vi "FFT Analysis (V1.24) 1.vi"() -> ()   [LabVIEW 2020]
uses:
  API/Generic Utilities_class/Generic Utilities.lvclass
  gSPWB.lvclass
  <vilib>/addons/_AddQ/G#Object/G#Object.lvclass
  API/GSwFormDSP_class/GSwFormDSP.lvclass
  API/GSwFormDSP_class/functions/Spectrum Display Options.ctl
  API/GSwFormDSP_class/functions/Attribute List.ctl
  C:/Program Files/National Instruments/LabVIEW 2020/vi.lib/addons/_AddQ/G#Object/G#Object.lvclass
  C:/Program Files/National Instruments/LabVIEW 2020/vi.lib/addons/_AddQ/IG#/IG#.lvclass
  C:/Users/fcharett/docsWork/coding/20openSourceSPWB/API/Generic Utilities_class/Generic Utilities.lvclass
  C:/Users/fcharett/docsWork/coding/20openSourceSPWB/API/GSwFormDSP_class/GSwFormDSP.lvclass
  SPWB.lvclass
  C:/Users/fcharett/docsWork/coding/20openSourceSPWB/SPWB_class/SPWB.lvclass
  API/GSwFormDSP_class/functions/Spectral Function Type.ctl
  <vilib>/Analysis/4window.llb/windowTd.ctl
  <vilib>/Analysis/NI_AALPro.lvlib
  API/GSwFormDSP_class/functions/Acoustic Weighting.ctl
panel:
  out "Version":string
  in  "Plot Names":string[](array[string])
  in  "Help":bool
  in  "wForms":waveform(dbl)[](array[waveform])
  in  "Exit":bool
  in  "reference in":refnum<class "SPWB.lvclass">
  out "PSD":waveform(dbl)[](array[waveform])
  in  "Signals selector":bool[](array[boolean])
  in  "DSP Functions":T1(tab)=enum."Spectral Analysis"
  in  "Load FROM File:":T2(ring)
  in  "Acoustic Weighting":T3
  in  "Spectrum Display Options":T4
  in  "Spectral Function Type":T5
  in  "Spectral Function Parameters - User":T7={"Frequency resolution (Hz)"=enum."1.0 Hz", "Overlap in %"=enum."0", "Window"=0} {"Window" items=["Rectangle"=0, "Hanning"=1, "Hamming"=2, "Blackman-Harris"=3, "Exact Blackman"=4, "Blackman"=5, "Flat Top"=6, "4 Term B-Harris "=7, "7 Term B-Harris"=8, "Low Sidelobe"=9, "Blackman Nuttall"=11, "Triangle"=30, "Bartlett-Hanning"=31, "Bohman"=32, "Parzen"=33, "Welch"=34, "Kaiser"=60, "Dolph-Chebyshev"=61, "Gaussian"=62]}
  in  "Average":enum16{"Select Here ...", "Energetic Average"}(ring)
  in  "Integrate":bool
  in  "Differentiate":bool
  in  "End Frequency (Hz)":dbl
  out "EB Result Table":string[][](table)
  in  "Start Frequency (Hz)":dbl
  in  "Export table to clipboard":bool
  in  "Import Signals":u16(ring) items=["Import Signals from another figure ..."]
  in  "Delete signals":bool
  in  "Graph":waveform(dbl)[](graph) caption="Waveform Graph"
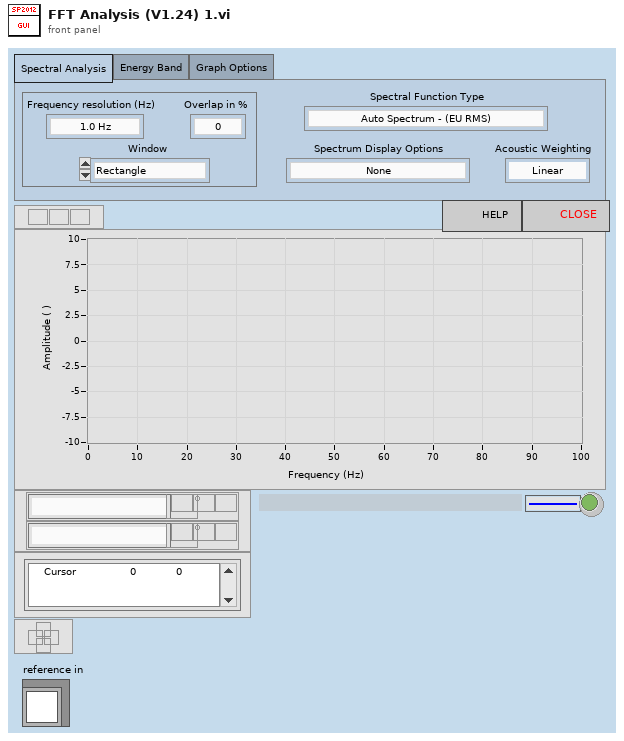
[diagram p1: front panel]
types:
  T1 = enum32{"File I/O", "Spectral Analysis", "Energy Band", "Graph Options"}
  T2 = enum16{"Click here to select ...", "LabView (*.tdms)", "RPC III (*.rsp)", "Wave Files (*.wav)", "Text Files (*.csv)", "MatLab - Test.Lab Export (*.mat)", "SSI Track Scan (*.erd, *.txt)", "LabView (*.fsigv2;*.fsigv1;*.swf)", "Prosig (*.dac)"}
  T3 = typedef "GSwFormDSP.lvclass/Acoustic Weighting.ctl" = enum16{"Linear", "A-weighting"}
  T4 = typedef "GSwFormDSP.lvclass/Spectrum Display Options.ctl" = enum16{"None", "dB - NO reference value", "dB - Automatic reference value", "dB - Sound SPL (ref 20E-6 Pa)", "dB - Acceleration (ref 1E-6 m/s²)", "dB - Velocity (ref 1E-9 m/s)", "dB - Displacement (ref 1E-12 m)"}
  T5 = typedef "GSwFormDSP.lvclass/Spectral Function Type.ctl" = enum16{"Auto Spectrum - (EU RMS)", "Auto Spectrum - (EU Peak)", "Power Spectrum - (EU RMS²)", "Power Spectrum - (EU Peak²)", "Auto Spectrum Density - (EU RMS/rtHz)", "Auto Spectrum Density - (EU Peak/rtHz)", "Power Spectrum Density - (EU RMS²/Hz)", "Power Spectrum Density - (EU Peak²/Hz)"}
  T6 = typedef "NI_AALPro.lvlib/windowTd.ctl" = u32
  T7 = cluster{"Frequency resolution (Hz)":enum16{"0.125 Hz", "0.25 Hz", "0.5 Hz", "1.0 Hz", "2.0 Hz", "4.0 Hz", "8.0 Hz", "16 Hz", "32 Hz", "64 Hz", "128 Hz"}, "Overlap in %":enum16{"0", "10", "20", "30", "40", "50", "60", "70", "80", "90"}, "Window":T6}
  T8 = typedef "GSwFormDSP.lvclass/Attribute List.ctl" = string
  T9 = enum16{"1 octave", "1/3 octave", "1/6 octave", "1/12 octave", "1/24 octave"}
  T10 = enum8{"Enabled", "Disabled", "Disabled and Grayed Out"}
  T11 = enum32{"Invalid", "Standard", "Closed", "Hidden", "Minimized", "Maximized"}
  T12 = enum16{"Always On", "Always Off", "Off While Running"}
  T13 = enum16{"Keep the full path", "File name ONLY", "Keep the full path - Force file name display"}
  T14 = cluster{"Color":u32, "PointStyle":u8, "LineStyle":u8, "Interp":u8, "LineWidth":u8, "BarPlotStyle":u8, "FillTo":i16, "XScaleIdx":u32, "YScaleIdx":u32, "Anti-Aliased":bool, "LabelFormat":u8, "TransitionType":u8, "TransitionLocation":u8, "DigitalLineStyle":u8}
  T15 = typedef "LVCursorListTypeDef.ctl" = cluster{"Name":string, "Color":u32, "Style":u8, "Point Style":u8, "Name Visible":bool, "Allow Drag":bool, "Cursor Mode":u32, "Plot":i32, "Index":i32, "Position":cluster{"X":dbl, "Y":dbl}, "X Scale":u32, "Y Scale":u32, "Watch Plots":i32[], "Watch All Plots":bool, "Plot Area":i32, "Label Offset":cluster{"X":dbl, "Y":dbl}}[]
  T16 = cluster{"Name":string, "Color":u32, "Style":u8, "Point Style":u8, "Name Visible":bool, "Allow Drag":bool, "Cursor Mode":u32, "Plot":i32, "Index":i32, "Position":cluster{"X":dbl, "Y":dbl}, "X Scale":u32, "Y Scale":u32, "Watch Plots":i32[], "Watch All Plots":bool, "Plot Area":i32, "Label Offset":cluster{"X":dbl, "Y":dbl}}
  T17 = cluster{"Window Name Index":string, "wForm Ref":refnum<class "GSwFormDSP.lvclass">}[]
  T18 = cluster{"Window Name Index":string, "wForm Ref":refnum<class "GSwFormDSP.lvclass">}
  T19 = typedef "LVRectTypeDef.ctl" = cluster{"Left":i16, "Top":i16, "Right":i16, "Bottom":i16}
  T20 = cluster{"Name":string, "Color":u32, "Style":u8, "Point Style":u8, "Name Visible":bool, "Allow Drag":bool, "Cursor Mode":u32, "Plot":i32, "Index":i32, "Position":cluster{"X":dbl, "Y":dbl}, "X Scale":u32, "Y Scale":u32, "Watch Plots":i32[], "Watch All Plots":bool, "Plot Area":i32, "Label Offset":cluster{"X":dbl, "Y":dbl}}[]
  T21 = cluster{"Window Name Index":string, "reference out":refnum<class "GSwFormDSP.lvclass">}
  T22 = cluster{"Window Name Index":string, "reference out":refnum<class "GSwFormDSP.lvclass">}[]
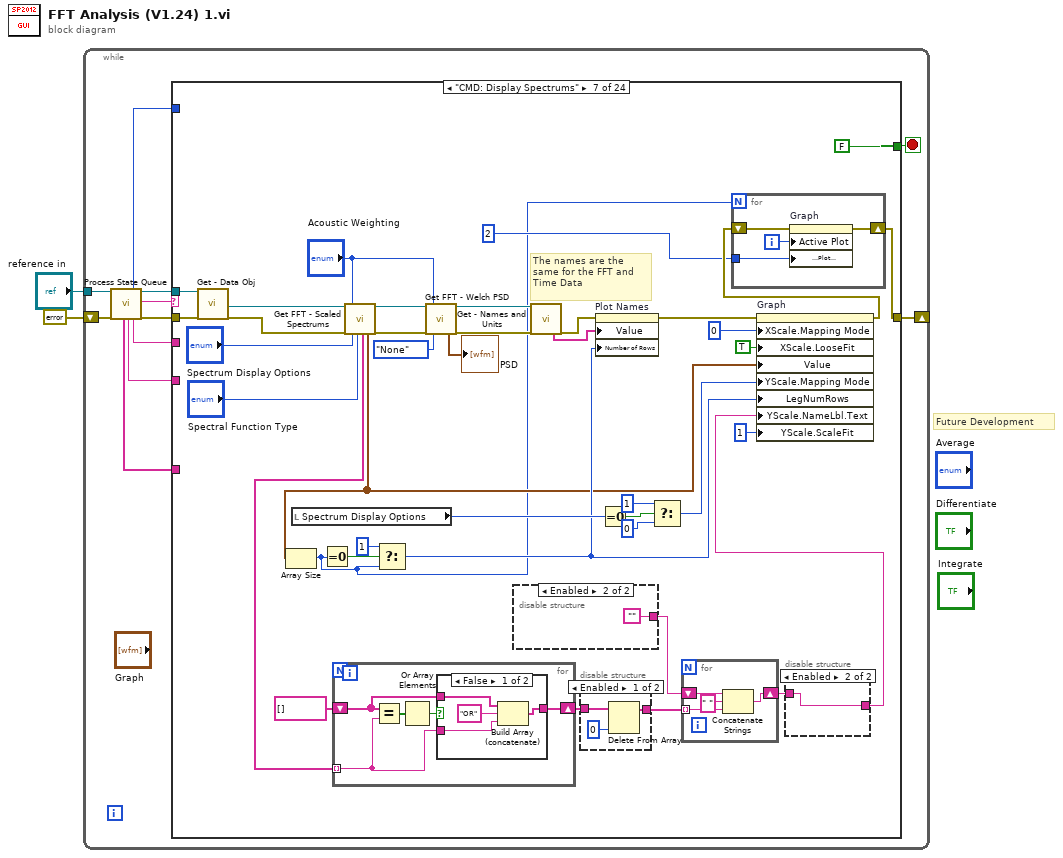
[diagram p0: block diagram]
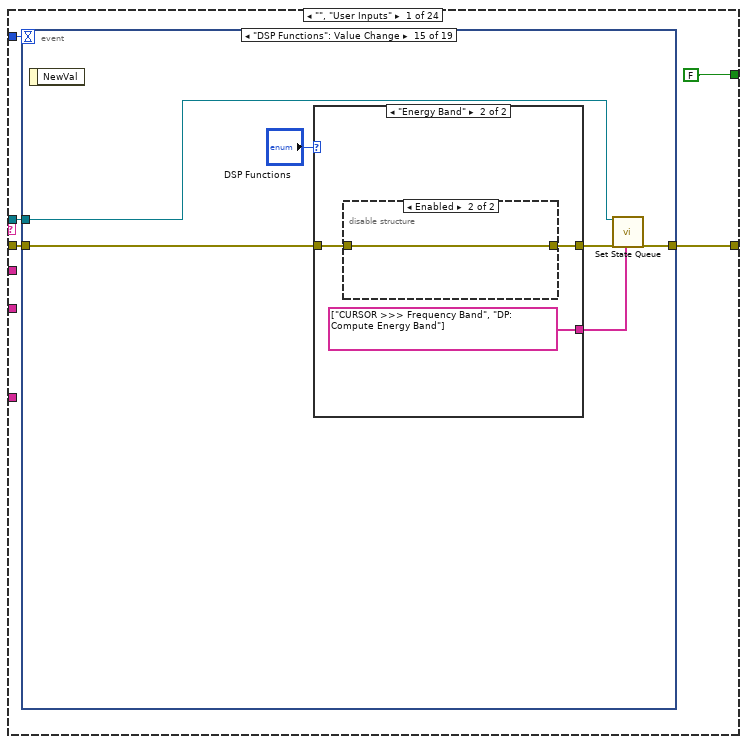
[diagram p2: hidden frame]
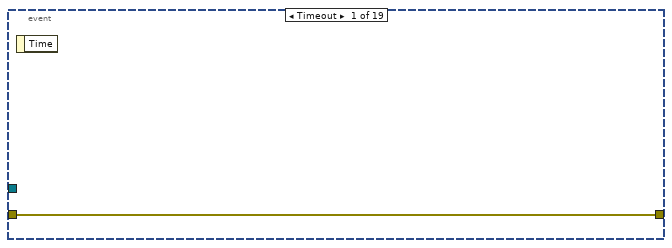
[diagram p3: hidden frame]
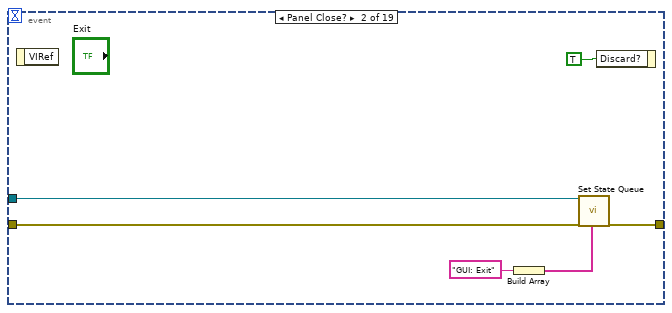
[diagram p4: hidden frame]
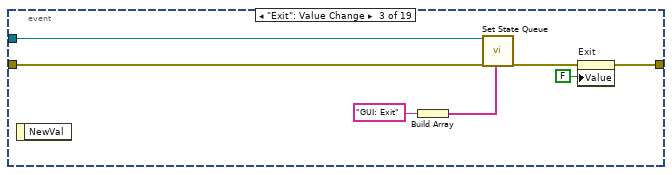
[diagram p5: hidden frame]
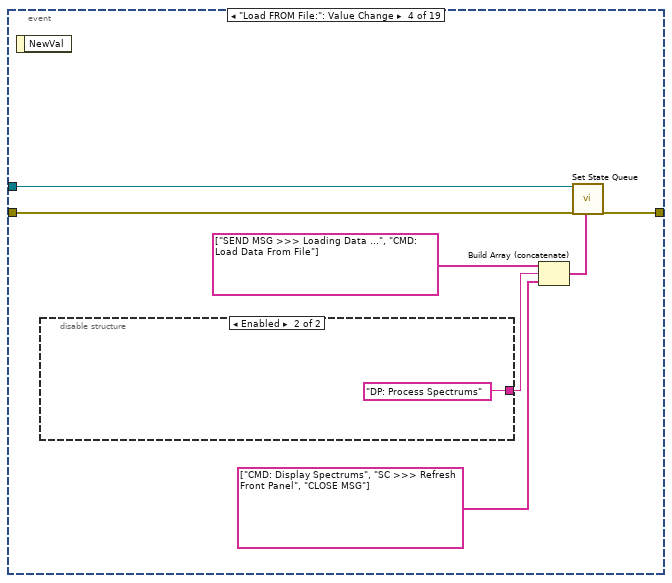
[diagram p6: hidden frame]
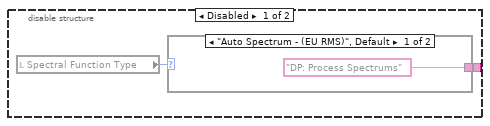
[diagram p7: hidden frame]
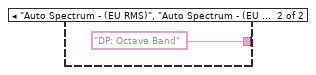
[diagram p8: hidden frame]
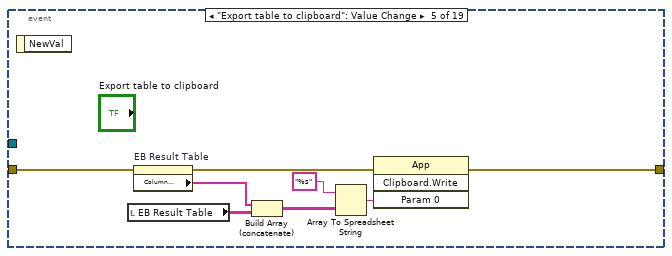
[diagram p9: hidden frame]
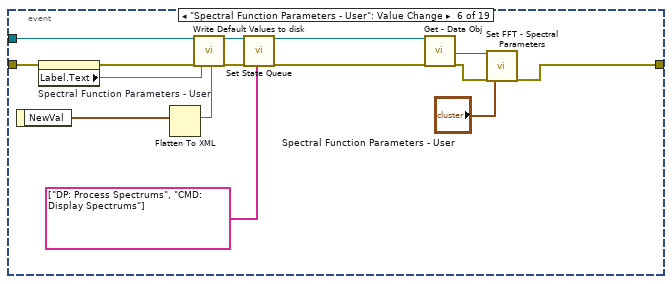
[diagram p10: hidden frame]
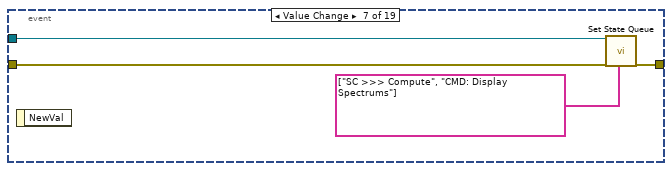
[diagram p11: hidden frame]
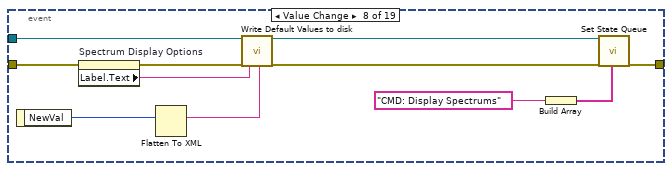
[diagram p12: hidden frame]
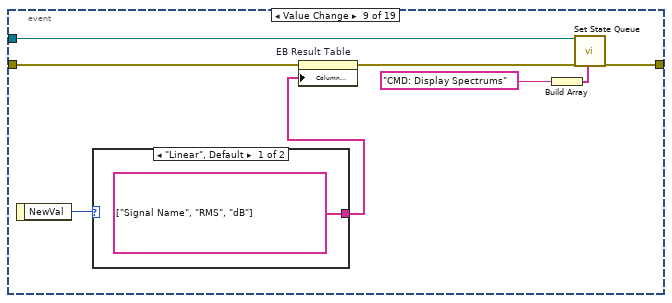
[diagram p13: hidden frame]
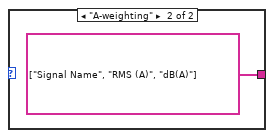
[diagram p14: hidden frame]
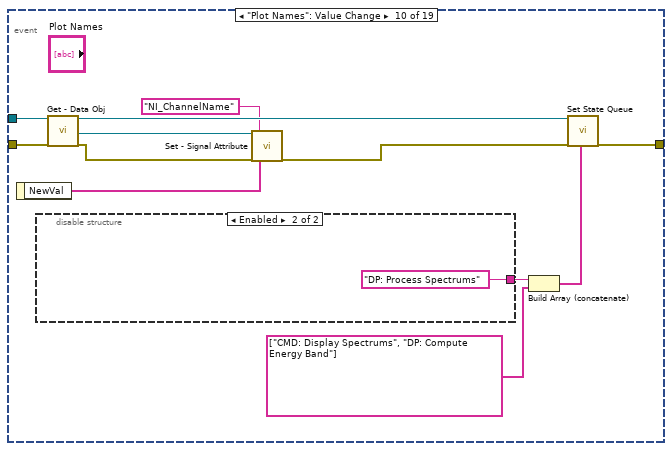
[diagram p15: hidden frame]
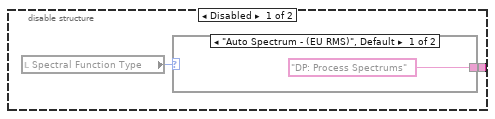
[diagram p16: hidden frame]
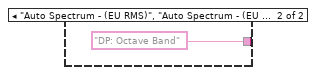
[diagram p17: hidden frame]
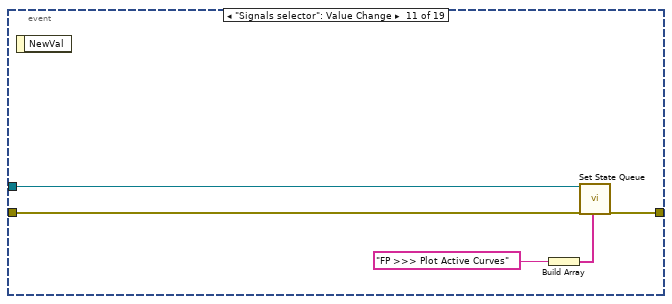
[diagram p18: hidden frame]
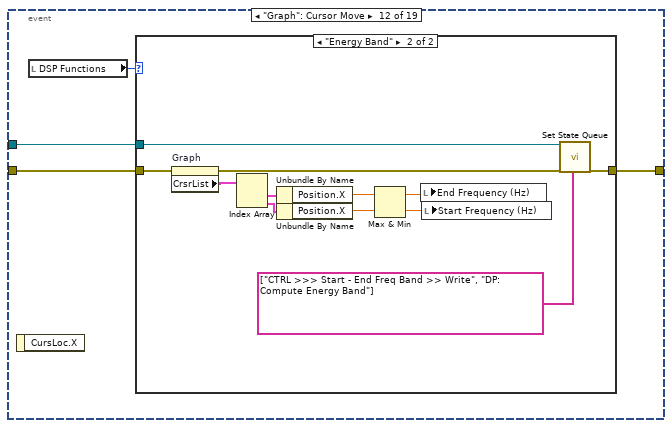
[diagram p19: hidden frame]
diagram:
  # "Future Development"
  n1 = while {
    shift-right: [w13] -> _
    shift-left: errorcluster {"status"=FALSE, "code"=0, "source"=""} ("error out") -> [w11]
    tunnel: "reference in" -> [w10]
    stop <- w12 stop-if-true
    n2 = call "Process State Queue.vi"("reference in"=w10, "error in (no error)"=w11) -> ("State History"=w3:string[], "Additional Options"=w4:string, "Timeout"=w7:i32, "State Option"=w5:string, "reference out"=w6:refnum<class "SPWB.lvclass">, "Current State"=w8:string, "error out"=w9:errorcluster)  [unwired: 10 in, 1 out]
    n3 = case shown="\"CMD: Display Spectrums\"" w8 {
      selector: w8 -> [_ _ _ _ _ _ _ _ _ _ _ _ _ _ _ _ _ _ _ _ w989 _ _ _]
      tunnel: w9 -> [w15 w299 w302 w322 w330 w367 w391 w437 w441 w448 w468 w472 w642 w801 w863 w880 w894 w943 w970 w985 w988 w997 w1007 w1009]
      tunnel: [w16 w299 w301 w320 w330 w367 w376 w438 w441 w446 w468 w473 w643 w802 w863 w876 w893 w942 w968 w985 w988 errorcluster {"status"=FALSE, "code"=0, "source"=""} ("error out") w1007 w1009] -> w13
      tunnel: [FALSE FALSE FALSE FALSE FALSE FALSE FALSE FALSE FALSE FALSE FALSE FALSE FALSE FALSE FALSE FALSE TRUE FALSE FALSE FALSE FALSE FALSE FALSE TRUE] -> w12
      tunnel: w7 -> [w17 _ _ _ _ _ _ _ _ _ _ _ _ _ _ _ _ _ _ _ _ _ _ _]
      tunnel: w6 -> [w14 _ w303 w321 _ _ w390 _ _ w447 _ w471 w640 _ _ w879 w895 w944 w969 _ _ _ _ _]
      tunnel: w5 -> [_ _ _ _ _ _ _ _ _ w443 _ w474 w641 w800 _ _ _ w945 _ _ _ _ _ _]
      tunnel: w4 -> [_ _ _ _ _ _ _ _ _ _ _ w470 w639 _ _ _ _ _ _ _ _ _ _ _]
      tunnel: w3 -> [_ _ _ _ _ _ _ _ _ _ _ _ _ _ _ _ _ _ _ _ _ w1000 _ _]
      frame "", "User Inputs" {
        n4 = event shown="[14] \"DSP Functions\": Value Change" {
          selector: _ -> [_ _ _ _ _ _ _ _ _ _ _ _ _ _ _ _ _ _ _]
          dyn-events: _ -> [_ _ _ _ _ _ _ _ _ _ _ _ _ _ _ _ _ _ _]
          timeout: w17 -> [_ _ _ _ _ _ _ _ _ _ _ _ _ _ _ _ _ _ _]
          tunnel: [w19 w21 w32 w38 w50 w57 w71 w73 w90 w97 w110 w116 w135 w144 w160 w180 w211 w284 w298] -> w16
          tunnel: w15 -> [w19 w22 w27 w39 w49 w55 w69 w82 w86 w102 w112 w117 w142 w147 w163 w186 w206 w287 w298]
          tunnel: w14 -> [_ w23 w28 w37 _ w66 w68 w81 w89 w103 w113 w115 w137 w146 w162 w187 w207 w261 _]
          event Timeout {
            n5 = event-data() -> ()  [unwired: 1 in, 1 out]
          }
          event Panel Close? {
            n6 = event-data() -> ()  [unwired: 1 in, 1 out]
            n7 = Build Array("GUI: Exit") -> (w20:string[])
            n8 = call "Set State Queue.vi"("reference in"=w23, "error in (no error)"=w22, "State Queue"=w20) -> ("error out"=w21:errorcluster)  [unwired: 15 in, 1 out]
            n9 = event-data("Discard?"=TRUE) -> ()  [unwired: 1 in, 1 out]
          }
          event "Exit": Value Change {
            n10 = event-data() -> ()  [unwired: 1 in, 1 out]
            n11 = Build Array("GUI: Exit") -> (w29:string[])
            n12 = call "Set State Queue.vi"("reference in"=w28, "error in (no error)"=w27, "State Queue"=w29) -> ("error out"=w26:errorcluster)  [unwired: 15 in, 1 out]
            n13 = property on="Exit" class="Bool (strict)"(error in=w26, "Value"=FALSE ("Exit")) -> (error out=w32:errorcluster)  [unwired: 1 in, 1 out]
          }
          event "Load FROM File:": Value Change {
            n14 = event-data() -> ()  [unwired: 1 in, 1 out]
            n15 = disable-structure shown="Enabled" {
              disable-tunnel: [w40 "DP: Process Spectrums" ("String")] -> w35
              frame Disabled {
                n16 = local read "Spectral Function Type"() -> (w41:T5)
                n17 = case shown="\"Auto Spectrum - (EU RMS)\", Default" w41 {
                  tunnel: ["DP: Process Spectrums" ("String") "DP: Octave Band" ("String")] -> w40
                  frame "Auto Spectrum - (EU RMS)", Default {
                  }
                  frame "Auto Spectrum - (EU RMS)", "Auto Spectrum - (EU Peak)" {
                  }
                }
              }
              frame Enabled {
              }
            }
            n18 = Build Array (concatenate)(string[] ["SEND MSG >>> Loading Data ...", "CMD: Load Data From File"] ("State Queue OUT"), w35, string[] ["CMD: Display Spectrums", "SC >>> Refresh Front Panel", "CLOSE MSG"] ("State Queue OUT")) -> (w33:string[])
            n19 = call "Set State Queue.vi"("reference in"=w37, "error in (no error)"=w39, "State Queue"=w33) -> ("error out"=w38:errorcluster)  [unwired: 15 in, 1 out]
          }
          event "Export table to clipboard": Value Change {
            n20 = event-data() -> ()  [unwired: 1 in, 1 out]
            n21 = local read "EB Result Table"() -> (w46:string[][])
            n22 = property on="EB Result Table" class="Tbl (strict)"(error in=w49) -> (error out=w48:errorcluster, "Column Headers[]"=w47:string[])  [unwired: 1 in, 1 out]
            n23 = Build Array (concatenate)(w47, w46) -> (w45:string[][])
            n24 = Array To Spreadsheet String(array=w45, 3:"%s" ("format string")) -> (spreadsheet string=w51:string)  [unwired: 1 in]
            n25 = invoke class="App" method="Clipboard.Write"(error in=w48, "Param 0"=w51) -> (error out=w50:errorcluster)  [unwired: 2 in, 3 out]
          }
          event "Spectral Function Parameters - User": Value Change {
            n26 = event-data() -> ("NewVal"=w67:T7)  [unwired: 1 in]
            n27 = property on="Spectral Function Parameters - User" class="Clust (strict)"(error in=w55) -> (error out=w54:errorcluster, "Label.Text"=w53:string)  [unwired: 1 in, 1 out]
            n28 = Flatten To XML(6:w67) -> (2:w65:string)
            n29 = call-dynamic "Write Default Values to disk.vi"("reference in"=w66, "error in (no error)"=w54, "Control Label"=w53, "Value (XML String)"=w65) -> ("reference out"=w63:refnum<class "SPWB.lvclass">, "error out"=w64:errorcluster)  [unwired: 14 in]
            n30 = call "Set State Queue.vi"("reference in"=w63, "error in (no error)"=w64, "State Queue"=string[] ["DP: Process Spectrums", "CMD: Display Spectrums"]) -> ("reference out"=w62:refnum<class "SPWB.lvclass">, "error out"=w61:errorcluster)  [unwired: 15 in]
            n31 = call "Get - Data Obj.vi"("reference in"=w62, "error in (no error)"=w61) -> ("Data"=w60:refnum<class "GSwFormDSP.lvclass">, "error out"=w59:errorcluster)  [unwired: 15 in, 1 out]
            n32 = call "Set FFT - Spectral Parameters.vi"("reference in"=w60, "error in (no error)"=w59, "Spectral Function Parameters - User"="Spectral Function Parameters - User") -> ("error out"=w57:errorcluster)  [unwired: 15 in, 1 out]
          }
          event Value Change {
            n33 = event-data() -> ()  [unwired: 1 in, 1 out]
            n34 = call "Set State Queue.vi"("reference in"=w68, "error in (no error)"=w69, "State Queue"=string[] ["SC >>> Compute", "CMD: Display Spectrums"]) -> ("error out"=w71:errorcluster)  [unwired: 15 in, 1 out]
          }
          event Value Change {
            n35 = event-data() -> ("NewVal"=w72:T4)  [unwired: 1 in]
            n36 = property on="Spectrum Display Options" class="Enum (strict)"(error in=w82) -> (error out=w80:errorcluster, "Label.Text"=w79:string)  [unwired: 1 in, 1 out]
            n37 = Flatten To XML(6:w72) -> (2:w78:string)
            n38 = call-dynamic "Write Default Values to disk.vi"("reference in"=w81, "error in (no error)"=w80, "Control Label"=w79, "Value (XML String)"=w78) -> ("reference out"=w77:refnum<class "SPWB.lvclass">, "error out"=w76:errorcluster)  [unwired: 14 in]
            n39 = Build Array("CMD: Display Spectrums") -> (w74:string[])
            n40 = call "Set State Queue.vi"("reference in"=w77, "error in (no error)"=w76, "State Queue"=w74) -> ("error out"=w73:errorcluster)  [unwired: 15 in, 1 out]
          }
          event Value Change {
            n41 = event-data() -> ("NewVal"=w84:T3)  [unwired: 1 in]
            n42 = case shown="\"Linear\", Default" w84 {
              tunnel: [string[] ["Signal Name", "RMS", "dB"] ("Column Header Strings[]") string[] ["Signal Name", "RMS (A)", "dB(A)"] ("Column Header Strings[]")] -> w83
              frame "Linear", Default {
              }
              frame "A-weighting" {
              }
            }
            n43 = property on="EB Result Table" class="Tbl (strict)"(error in=w86, "Column Headers[]"=w83) -> (error out=w85:errorcluster)  [unwired: 1 in, 1 out]
            n44 = Build Array("CMD: Display Spectrums") -> (w87:string[])
            n45 = call "Set State Queue.vi"("reference in"=w89, "error in (no error)"=w85, "State Queue"=w87) -> ("error out"=w90:errorcluster)  [unwired: 15 in, 1 out]
          }
          event "Plot Names": Value Change {
            n46 = event-data() -> ("NewVal"=w104:string[])  [unwired: 1 in]
            n47 = disable-structure shown="Enabled" {
              disable-tunnel: [w105 "DP: Process Spectrums" ("String")] -> w96
              frame Disabled {
                n48 = local read "Spectral Function Type"() -> (w106:T5)
                n49 = case shown="\"Auto Spectrum - (EU RMS)\", Default" w106 {
                  tunnel: ["DP: Process Spectrums" ("String") "DP: Octave Band" ("String")] -> w105
                  frame "Auto Spectrum - (EU RMS)", Default {
                  }
                  frame "Auto Spectrum - (EU RMS)", "Auto Spectrum - (EU Peak)" {
                  }
                }
              }
              frame Enabled {
              }
            }
            n50 = call "Get - Data Obj.vi"("reference in"=w103, "error in (no error)"=w102) -> ("reference out"=w99:refnum<class "gSPWB.lvclass">, "Data"=w100:refnum<class "GSwFormDSP.lvclass">, "error out"=w101:errorcluster)  [unwired: 15 in]
            n51 = call-dynamic "Set - Signal Attribute.vi"("reference in"=w100, "error in (no error)"=w101, "wForm Attributes"=T8 "NI_ChannelName", "Attribute"=w104) -> ("error out"=w98:errorcluster)  [unwired: 14 in, 1 out]
            n52 = Build Array (concatenate)(w96, string[] ["CMD: Display Spectrums", "DP: Compute Energy Band"]) -> (w94:string[])
            n53 = call "Set State Queue.vi"("reference in"=w99, "error in (no error)"=w98, "State Queue"=w94) -> ("error out"=w97:errorcluster)  [unwired: 15 in, 1 out]
          }
          event "Signals selector": Value Change {
            n54 = event-data() -> ()  [unwired: 1 in, 1 out]
            n55 = Build Array("FP >>> Plot Active Curves") -> (w111:string[])
            n56 = call "Set State Queue.vi"("reference in"=w113, "error in (no error)"=w112, "State Queue"=w111) -> ("error out"=w110:errorcluster)  [unwired: 15 in, 1 out]
          }
          event "Graph": Cursor Move {
            n57 = event-data() -> ()  [unwired: 1 in, 1 out]
            n58 = local read "DSP Functions"() -> (w118:T1)
            n59 = case shown="\"Energy Band\"" w118 {
              tunnel: w117 -> [w119 w131]
              tunnel: [w119 w122] -> w116
              tunnel: w115 -> [_ w121]
              frame "File I/O", Default {
                # "Do NOT do anything if we are NOT in energy band mode."
              }
              frame "Energy Band" {
                n60 = property on="Graph" class="WFGraph (strict)"(error in=w131) -> (error out=w120:errorcluster, "CrsrList"=w130:T15)  [unwired: 1 in, 1 out]
                n61 = Index Array(array=w130) -> (element #1=w129:T16, element #2=w128:T16)  [unwired: 2 in]
                n62 = Unbundle By Name(w129) -> ("Position.X"=w127:dbl)
                n63 = Unbundle By Name(w128) -> ("Position.X"=w126:dbl)
                n64 = Max & Min(x=w127, y=w126) -> (max(x,y)=w124:dbl, min(x,y)=w125:dbl)
                n65 = local write "End Frequency (Hz)"(w124) -> ()
                n66 = local write "Start Frequency (Hz)"(w125) -> ()
                n67 = call "Set State Queue.vi"("reference in"=w121, "error in (no error)"=w120, "State Queue"=string[] ["CTRL >>> Start - End Freq Band >> Write", "DP: Compute Energy Band"]) -> ("error out"=w122:errorcluster)  [unwired: 15 in, 1 out]
              }
            }
          }
          event "Graph": Plot Attribute Change {
            n68 = event-data() -> ("PlotIdx"=w140:i32, "NewAttrib"=w138:T14)  [unwired: 1 in]
            n69 = property on="Graph" class="WFGraph (strict)"(error in=w142) -> (error out=w136:errorcluster, "Label.Text"=w134:string)  [unwired: 1 in, 1 out]
            n70 = Number To Decimal String(number=w140) -> (decimal integer string=w139:string)  [unwired: 1 in]
            n71 = Flatten To XML(6:w138) -> (2:w132:string)
            n72 = Concatenate Strings("Plot " ("string"), w139) -> (w133:string)
            n73 = call-dynamic "Write Default Values to disk.vi"("reference in"=w137, "error in (no error)"=w136, "Control Label"=w134, "Caption"=w133, "Value (XML String)"=w132) -> ("error out"=w135:errorcluster)  [unwired: 13 in, 1 out]
          }
          event "Start Frequency (Hz)", "End Frequency (Hz)": Value Change {
            n74 = event-data() -> ()  [unwired: 1 in, 1 out]
            n75 = Greater?(x="Start Frequency (Hz)", y="End Frequency (Hz)") -> (0:w154:bool)
            n76 = case shown="True" w154 {
              tunnel: "End Frequency (Hz)" -> [w155 w158]
              tunnel: "Start Frequency (Hz)" -> [w156 w157]
              tunnel: [w156 w158] -> w150
              tunnel: [w155 w157] -> w148
              frame False {
              }
              frame True {
                # "The Start frequency is higher than the End, so swap the values!"
                n77 = local write "End Frequency (Hz)"(w157) -> ()
                n78 = local write "Start Frequency (Hz)"(w158) -> ()
              }
            }
            n79 = property on="Graph" class="WFGraph (strict)"(error in=w147, "Active Cursor"=u32 0, "Cursor.Cursor X"=w150, "Active Cursor"=u32 1, "Cursor.Cursor X"=w148) -> (error out=w145:errorcluster)  [unwired: 1 in, 1 out]
            n80 = call "Set State Queue.vi"("reference in"=w146, "error in (no error)"=w145, "State Queue"=string[] ["CTRL >>> Start - End Freq Band >> Write", "DP: Compute Energy Band"]) -> ("error out"=w144:errorcluster)  [unwired: 15 in, 1 out]
          }
          event "DSP Functions": Value Change {
            n81 = event-data() -> ()  [unwired: 1 in, 1 out]
            n82 = case shown="\"Energy Band\"" "DSP Functions" {
              tunnel: w163 -> [w167 w170]
              tunnel: [w167 w169] -> w161
              tunnel: [w166 string[] ["CURSOR >>> Frequency Band", "DP: Compute Energy Band"] ("appended array")] -> w159
              frame "File I/O", Default {
                n83 = Build Array("CURSOR >>> Default") -> (w166:string[])
              }
              frame "Energy Band" {
                n84 = disable-structure shown="Enabled" {
                  disable-tunnel: w170 -> [w175 w176]
                  disable-tunnel: [w173 w176] -> w169
                  frame Disabled {
                    n85 = property on="Graph" class="WFGraph (strict)"(error in=w175, "Active Cursor"=u32 0) -> (error out=w172:errorcluster, "Cursor.Cursor X"=w171:dbl)  [unwired: 1 in, 1 out]
                    n86 = property on="Start Frequency (Hz)" class="DigNum (strict)"(error in=w172, "Val(Sgnl)"=w171) -> (error out=w173:errorcluster)  [unwired: 1 in, 1 out]
                  }
                  frame Enabled {
                  }
                }
              }
            }
            n87 = call "Set State Queue.vi"("reference in"=w162, "error in (no error)"=w161, "State Queue"=w159) -> ("error out"=w160:errorcluster)  [unwired: 15 in, 1 out]
          }
          event "Delete signals": Value Change {
            n88 = event-data() -> ()  [unwired: 1 in, 1 out]
            n89 = local read "Signals selector"() -> (w189:bool[])
            n90 = disable-structure shown="Enabled" {
              disable-tunnel: [w190 "DP: Process Spectrums" ("String")] -> w179
              frame Disabled {
                n91 = local read "Spectral Function Type"() -> (w191:T5)
                n92 = case shown="\"Auto Spectrum - (EU RMS)\", Default" w191 {
                  tunnel: ["DP: Process Spectrums" ("String") "DP: Octave Band" ("String")] -> w190
                  frame "Auto Spectrum - (EU RMS)", Default {
                  }
                  frame "Auto Spectrum - (EU RMS)", "Auto Spectrum - (EU Peak)" {
                  }
                }
              }
              frame Enabled {
              }
            }
            n93 = for {
              shift-right: [w195] -> w183
              shift-left: i32[] [] -> [w196]
              tunnel: w189 -> [w198] mode=indexing
              i -> [w197]
              n94 = case shown="True" w198 {
                tunnel: w197 -> [_ w202]
                tunnel: w196 -> [w199 w201]
                tunnel: [w199 w200] -> w195
                frame False {
                }
                frame True {
                  n95 = Build Array (concatenate)(w201, w202) -> (w200:i32[])
                }
              }
            }
            n96 = call "Get - Data Obj.vi"("reference in"=w187, "error in (no error)"=w186) -> ("reference out"=w182:refnum<class "gSPWB.lvclass">, "Data"=w185:refnum<class "GSwFormDSP.lvclass">, "error out"=w184:errorcluster)  [unwired: 15 in]
            n97 = call "Set - Keep Specific Signals Delete the Rest.vi"("reference in"=w185, "error in (no error)"=w184, "Channels Index to KEEP"=w183) -> ("error out"=w181:errorcluster)  [unwired: 15 in, 1 out]
            n98 = Build Array (concatenate)(w179, string[] ["CMD: Display Spectrums", "SC >>> Refresh Front Panel"]) -> (w177:string[])
            n99 = call "Set State Queue.vi"("reference in"=w182, "error in (no error)"=w181, "State Queue"=w177) -> ("error out"=w180:errorcluster)  [unwired: 15 in, 1 out]
          }
          event "Import Signals": Mouse Enter {
            n100 = event-data() -> ()  [unwired: 1 in, 1 out]
            n101 = call "GetClass - Window Info.vi"("error in (no error)"=w206) -> ("Window Info"=w204:T17, "error out"=w208:errorcluster)  [unwired: 17 in]
            n102 = call "Get - Window Name Index.vi"("reference in"=w207, "error in (no error)"=w208) -> ("Window Name Index"=w205:string, "error out"=w203:errorcluster)  [unwired: 15 in, 1 out]
            n103 = for {
              tunnel: w204 -> [w220] mode=indexing
              shift-right: [w217] -> w214
              shift-left: string[] [] -> [w216]
              tunnel: w205 -> [w221]
              shift-right: [w218] -> w210
              shift-left: w203 -> [w219]
              n104 = Unbundle By Name(w220) -> ("Window Name Index"=w215:string)
              n105 = String Subset(string=w215, length (rest)=3 ("length (rest)")) -> (substring=w222:string)  [unwired: 1 in]
              n106 = case shown="\"FFT\", \"TDP\"" w222 {
                tunnel: w215 -> [_ w234]
                tunnel: w221 -> [_ w233]
                tunnel: w220 -> [_ w231]
                tunnel: w219 -> [w224 w230]
                tunnel: [w224 w229] -> w218
                tunnel: w215 -> [_ w228]
                tunnel: [w225 w227] -> w217
                tunnel: w216 -> [w225 w226]
                frame "", Default {
                }
                frame "FFT", "TDP" {
                  n107 = Equal?(x=w233, y=w234) -> (x = y?=w232:bool)
                  n108 = case shown="False" w232 {
                    tunnel: w231 -> [w243 _]
                    tunnel: w230 -> [w237 w249]
                    tunnel: [w236 w249] -> w229
                    tunnel: w228 -> [w242 _]
                    tunnel: [w241 w248] -> w227
                    tunnel: w226 -> [w239 w248]
                    frame False {
                      n109 = Unbundle By Name(w243) -> ("wForm Ref"=w238:refnum<class "GSwFormDSP.lvclass">)
                      n110 = call-dynamic "Get - Names and Units.vi"("reference in"=w238, "error in (no error)"=w237) -> ("Signal Names"=w235:string[], "error out"=w236:errorcluster)  [unwired: 13 in, 3 out]
                      n111 = for {
                        tunnel: w242 -> [w247]
                        tunnel: w235 -> [w245] mode=indexing
                        tunnel: [w244] -> w240 mode=indexing
                        n112 = Concatenate Strings(w247, " => " ("string"), w245) -> (w244:string)
                      }
                      n113 = Build Array (concatenate)(w239, w240) -> (w241:string[])
                    }
                    frame True {
                      # "This is the current window, do so nothing"
                    }
                  }
                }
              }
            }
            n114 = Build Array (concatenate)("Import Signals from another figure ..." ("string"), w214) -> (w209:string[])
            n115 = property on="Import Signals" class="Ring (strict)"(error in=w210, "Strings []"=w209) -> (error out=w211:errorcluster)  [unwired: 1 in, 1 out]
          }
          event "Import Signals": Value Change {
            n116 = event-data() -> ("NewVal"=w285:u16)  [unwired: 1 in]
            n117 = disable-structure shown="Enabled" {
              disable-tunnel: [w290 "DP: Process Spectrums" ("String")] -> w258
              frame Disabled {
                n118 = local read "Spectral Function Type"() -> (w291:T5)
                n119 = case shown="\"Auto Spectrum - (EU RMS)\", Default" w291 {
                  tunnel: ["DP: Process Spectrums" ("String") "DP: Octave Band" ("String")] -> w290
                  frame "Auto Spectrum - (EU RMS)", Default {
                  }
                  frame "Auto Spectrum - (EU RMS)", "Auto Spectrum - (EU Peak)" {
                  }
                }
              }
              frame Enabled {
              }
            }
            n120 = property on="Import Signals" class="Ring (strict)"(error in=w287) -> (error out=w273:errorcluster, "Strings []"=w286:string[])  [unwired: 1 in, 1 out]
            n121 = call "GetClass - Window Info.vi"("error in (no error)"=w273) -> ("Window Info"=w272:T17, "error out"=w270:errorcluster)  [unwired: 17 in]
            n122 = Index Array(array=w286, index=w285) -> (element=w288:string)
            n123 = for {
              tunnel: w272 -> [w296] mode=indexing
              tunnel: [w295] -> w282 mode=indexing
              n124 = Unbundle By Name(w296) -> ("Window Name Index"=w295:string)
            }
            n125 = Match Pattern(string=w288, regular expression=" => " ("string")) -> (before substring=w264:string, after substring=w277:string)  [unwired: 1 in, 2 out]
            n126 = Concatenate Strings(w277, " (" ("string"), w264, ")" ("string")) -> (w274:string)
            n127 = Search 1D Array(1D array=w282, element=w264) -> (index of element=w283:i32)  [unwired: 1 in]
            n128 = Index Array(array=w272, index=w283) -> (element=w280:T18)
            n129 = Unbundle By Name(w280) -> ("wForm Ref"=w271:refnum<class "GSwFormDSP.lvclass">)
            n130 = call-dynamic "Get - Names and Units.vi"("reference in"=w271, "error in (no error)"=w270) -> ("Signal Names"=w269:string[], "reference out"=w256:refnum<class "GSwFormDSP.lvclass">, "error out"=w255:errorcluster)  [unwired: 13 in, 2 out]
            n131 = Search 1D Array(1D array=w269, element=w277) -> (index of element=w253:i32)  [unwired: 1 in]
            n132 = Build Array(w253) -> (w252:i32[])
            n133 = call-dynamic "Get - wForms.vi"("reference in"=w256, "error in (no error)"=w255, "Indexes (Empty = ALL)"=w252) -> ("wForms"=w251:waveform(dbl)[], "error out"=w254:errorcluster)  [unwired: 13 in, 2 out]
            n134 = Index Array(array=w251) -> (element=w250:waveform(dbl))  [unwired: 1 in]
            n135 = Build Array (concatenate)(w258, string[] ["CMD: Display Spectrums", "SC >>> Refresh Front Panel"] ("State Queue OUT")) -> (w257:string[])
            n136 = Set Waveform Attribute(4:w254, 5:w274, 6:"NI_ChannelName" ("Att - wform Name"), 7:w250) -> (0:w262:errorcluster, 3:w279:waveform(dbl))  [unwired: 1 out]
            n137 = call "Get - Data Obj.vi"("reference in"=w261, "error in (no error)"=w262) -> ("reference out"=w265:refnum<class "gSPWB.lvclass">, "Data"=w266:refnum<class "GSwFormDSP.lvclass">, "error out"=w267:errorcluster)  [unwired: 15 in]
            n138 = Build Array(w279) -> (w260:waveform(dbl)[])
            n139 = call "Set - Append Signals to wForm.vi"("reference in"=w266, "error in (no error)"=w267, "New Signals"=w260) -> ("error out"=w268:errorcluster)  [unwired: 15 in, 1 out]
            n140 = call "Set State Queue.vi"("reference in"=w265, "error in (no error)"=w268, "State Queue"=w257) -> ("error out"=w263:errorcluster)  [unwired: 15 in, 1 out]
            n141 = property on="Import Signals" class="Ring (strict)"(error in=w263, "Value"=0) -> (error out=w284:errorcluster)  [unwired: 1 in, 1 out]
          }
          event "Help": Value Change {
            n142 = event-data() -> ()  [unwired: 1 in, 1 out]
            n143 = Control Help Window(1:TRUE ("Show")) -> ()  [unwired: 1 in]
          }
        }
      }
      frame "---- Data Processing ----" {
      }
      frame "DP: Octave Band" {
        n144 = disable-structure shown="Enabled" {
          disable-tunnel: w303 -> [w311 _]
          disable-tunnel: w302 -> [w310 w317]
          disable-tunnel: [w307 w317] -> w301
          frame Disabled {
            n145 = call "Get - Data Obj.vi"("reference in"=w311, "error in (no error)"=w310) -> ("Data"=w309:refnum<class "GSwFormDSP.lvclass">, "error out"=w308:errorcluster)  [unwired: 15 in, 1 out]
            n146 = local read "Spectral Function Type"() -> (w305:T5)
            n147 = case shown="\"1/3 Octave - (EU RMS)\"" w305 {
              tunnel: [T9."1 octave" ("Octave Bandwidth") T9."1/3 octave" ("Octave Bandwidth") T9."1/6 octave" ("Octave Bandwidth") T9."1/12 octave" ("Octave Bandwidth") T9."1/24 octave" ("Octave Bandwidth")] -> w306
              frame "Auto Spectrum Density - (EU RMS/rtHz)", Default {
              }
              frame "Power Spectrum - (EU RMS²)" {
              }
              frame "Power Spectrum - (EU Peak²)" {
              }
              frame "Auto Spectrum - (EU RMS)" {
              }
              frame "Auto Spectrum - (EU Peak)" {
              }
            }
            n148 = call "OCT - Auto Power Spectrums.vi"("reference in"=w309, "error in (no error)"=w308, "Octave Bandwidth"=w306) -> ("error out"=w307:errorcluster)  [unwired: 15 in, 1 out]
          }
          frame Enabled {
          }
        }
      }
      frame "DP: Process Spectrums" {
        n149 = call "Get - Data Obj.vi"("reference in"=w321, "error in (no error)"=w322) -> ("Data"=w318:refnum<class "GSwFormDSP.lvclass">, "error out"=w319:errorcluster)  [unwired: 15 in, 1 out]
        n150 = call "FFT - Auto Power Spectrums.vi"("reference in"=w318, "error in (no error)"=w319) -> ("error out"=w320:errorcluster)  [unwired: 15 in, 2 out]
      }
      frame "DP: Compute Energy Band" {
        # "The PSD is divided by the spectrum COMPLETE Lenght, not just the summation section!"
        n151 = local read "Start Frequency (Hz)"() -> (w329:dbl)
        n152 = local read "End Frequency (Hz)"() -> (w328:dbl)
        n153 = local read "Spectrum Display Options"() -> (w324:T4)
        n154 = local read "PSD"() -> (w331:waveform(dbl)[])
        n155 = Max & Min(x=w329, y=w328) -> (max(x,y)=w326:dbl, min(x,y)=w327:dbl)
        n156 = for {
          tunnel: w331 -> [w366] mode=indexing
          tunnel: w327 -> [w364]
          tunnel: w326 -> [w362]
          tunnel: [w354] -> w325 mode=indexing
          tunnel: w324 -> [w338]
          n157 = Unbundle By Name(w366) -> ("Y"=w359:dbl[], "dt"=w347:dbl)
          n158 = Divide(x=w364, y=w347) -> (x/y=w363:dbl)
          n159 = Divide(x=w362, y=w347) -> (x/y=w361:dbl)
          n160 = Array Size(array=w359) -> (size(s)=w358:i32)
          n161 = Round To Nearest(number=w363) -> (nearest integer value=w350:dbl)
          n162 = Round To Nearest(number=w361) -> (nearest integer value=w346:dbl)
          n163 = To Long Integer(number=w346) -> (32bit integer=w360:i32)
          n164 = Decrement(x=w358) -> (x-1=w356:i32)
          n165 = To Long Integer(number=w350) -> (32bit integer=w344:i32)
          n166 = Get Waveform Attribute(5:"unknown", 6:T8 "NI_ChannelName" ("wForm Attributes"), 7:w366) -> (1:w357:string, 3:w337:waveform(dbl))  [unwired: 1 in, 2 out]
          n167 = To Double Precision Float(number=w356) -> (double precision float=w351:dbl)
          n168 = Subtract(x=w360, y=w344) -> (x-y=w345:i32)
          n169 = Array Subset(array=w359, index=w344, length=w345) -> (w343:dbl[])
          n170 = Get Waveform Attribute(5:"", 6:T8 "NI_UnitDescription" ("wForm Attributes"), 7:w337) -> (1:w335:string)  [unwired: 1 in, 3 out]
          n171 = Add Array Elements(numeric array=w343) -> (sum=w353:dbl)
          n172 = Divide(x=w353, y=w351) -> (x/y=w352:dbl)
          n173 = Multiply(x=w350, y=w347) -> (x*y=w348:dbl)
          n174 = Multiply(x=w347, y=w346) -> (x*y=w349:dbl)
          n175 = Square Root(x=w352) -> (sqrt(x)=w342:dbl)
          n176 = local write "Start Frequency (Hz)"(w348) -> ()
          n177 = local write "End Frequency (Hz)"(w349) -> ()
          n178 = Number To Exponential String(number=w342) -> (E-format string=w355:string)  [unwired: 3 in]
          n179 = call "FFT - Compute dB Level - Single value.vi"("RMS EU Value"=w342, "Unit"=w335, "Spectrum Display Options"=w338) -> ("dB Value"=w341:dbl)  [unwired: 16 in]
          n180 = Number To Fractional String(number=w341, precision (6)=i16 2) -> (F-format string=w339:string)  [unwired: 2 in]
          n181 = Build Array(w357, w355, w339) -> (w354:string[])
        }
        "EB Result Table" <- w325
      }
      frame "---- Command ----" {
      }
      frame "CMD: Display Spectrums" {
        # "The names are the same for the FFT and Time Data"
        n182 = call "Get - Data Obj.vi"("reference in"=w390, "error in (no error)"=w391) -> ("Data"=w389:refnum<class "GSwFormDSP.lvclass">, "error out"=w388:errorcluster)  [unwired: 15 in, 1 out]
        n183 = local read "Spectrum Display Options"() -> (w399:T4)
        n184 = call "Get FFT - Scaled Spectrums.vi"("reference in"=w389, "error in (no error)"=w388, "Acoustic Weighting"="Acoustic Weighting", "Spectrum Display Options"="Spectrum Display Options", "Spectral Function Type"="Spectral Function Type") -> ("Spectrum Unit"=w384:string[], "Scaled Spectrums"=w385:waveform(dbl)[], "reference out"=w372:refnum<class "GSwFormDSP.lvclass">, "error out"=w371:errorcluster)  [unwired: 11 in]
        n185 = Array Size(array=w385) -> (size(s)=w374:i32)
        n186 = Equal To 0?(x=w374) -> (x = 0?=w401:bool)
        n187 = for {
          shift-right: [w429] -> w407
          shift-left: string[] [] -> [w428]
          tunnel: w384 -> [w427] mode=indexing
          n188 = Equal?(x=w428, y=w427) -> (x = y?=w431:bool[])
          n189 = Or Array Elements(Boolean array=w431) -> (logical OR=w430:bool)
          n190 = case shown="False" w430 {
            tunnel: [w434 w436] -> w429
            tunnel: w428 -> [w435 w436]
            tunnel: w427 -> [w433 _]
            frame False {
              n191 = Build Array (concatenate)(w435, "OR", w433) -> (w434:string[])
            }
            frame True {
            }
          }
        }
        n192 = Select(t=1, s=w401, f=w374) -> (s? t:f=w392:i32)
        n193 = call "Get FFT - Welch PSD.vi"("reference in"=w372, "error in (no error)"=w371, "Acoustic Weighting"="Acoustic Weighting", "Spectrum Display Options"=Spectrum_Display_Options."None") -> ("Welch PSD"=→"PSD":waveform(dbl)[], "reference out"=w382:refnum<class "GSwFormDSP.lvclass">, "error out"=w381:errorcluster)  [unwired: 13 in]
        n194 = disable-structure shown="Enabled" {
          disable-tunnel: ["Amplitude (" ""] -> w405
          frame Disabled {
          }
          frame Enabled {
          }
        }
        n195 = call-dynamic "Get - Names and Units.vi"("reference in"=w382, "error in (no error)"=w381) -> ("Signal Names"=w379:string[], "error out"=w380:errorcluster)  [unwired: 13 in, 3 out]
        n196 = disable-structure shown="Enabled" {
          disable-tunnel: [w420 w422] -> w406
          disable-tunnel: w407 -> [w419 w422]
          frame Enabled {
            n197 = Delete From Array(array=w419, index=0) -> (array with subset deleted=w420:string[])  [unwired: 1 in, 1 out]
          }
          frame Disabled {
          }
        }
        n198 = property on="Plot Names" class="Arr (strict)"(error in=w380, "Value"=w379, "Number of Rows"=w392) -> (error out=w393:errorcluster)  [unwired: 1 in, 1 out]
        n199 = Equal To 0?(x=w399) -> (x = 0?=w398:bool)
        n200 = Select(t=u8 1 ("Y Scale.Mapping Mode"), s=w398, f=u8 0 ("Y Scale.Mapping Mode")) -> (s? t:f=w395:u8)
        n201 = for {
          shift-right: [w423] -> w403
          shift-left: w405 -> [w426]
          tunnel: w406 -> [w425] mode=indexing
          n202 = Concatenate Strings(w426, " ", w425) -> (w423:string)
        }
        n203 = disable-structure shown="Enabled" {
          disable-tunnel: w403 -> [w416 w418]
          disable-tunnel: [w415 w418] -> w400
          frame Disabled {
            n204 = Concatenate Strings(w416, " )" ("string")) -> (w415:string)
          }
          frame Enabled {
          }
        }
        n205 = property on="Graph" class="WFGraph (strict)"(error in=w393, "XScale.Mapping Mode"=u8 0 ("Plot.Plot Interpolation"), "XScale.LooseFit"=TRUE ("X Scale.Loose Fit"), "Value"=w385, "YScale.Mapping Mode"=w395, "LegNumRows"=w392, "YScale.NameLbl.Text"=w400, "YScale.ScaleFit"=u8 1 ("Y Scale.Scale Fit")) -> (error out=w377:errorcluster)  [unwired: 1 in, 1 out]
        n206 = for {
          N: w374 -> [_]
          shift-right: [w410] -> w376
          shift-left: w377 -> [w411]
          tunnel: u8 2 ("Plot.Plot Interpolation") -> [w409]
          i -> [w412]
          n207 = property on="Graph" class="WFGraph (strict)"(error in=w411, "Active Plot"=w412, "Plot.Plot Interpolation"=w409) -> (error out=w410:errorcluster)  [unwired: 1 in, 1 out]
        }
      }
      frame "CMD: Load Data From File" {
        n208 = property on="Load FROM File:" class="Enum (strict)"(error in=w437, "Value"=0) -> (error out=w438:errorcluster)  [unwired: 1 in, 1 out]
      }
      frame "---- Scripts ----" {
      }
      frame "SC" {
        n209 = case shown="\"Initialize\", Default" w443 {
          tunnel: [string[] ["GUI: Initialize Ref", "FP >>> Default Panel Position and Size", "CTRL >>> Spectral Function Parameters ", "CTRL >>> Spectral Function Type", "CTRL >>> Spectrum Display Options", "CTRL >>> Version Number", "CTRL >>> DSP Function", "CTRL >>> Start - End Freq Band >> Read", "SC >>> Compute", "CMD: Display Spectrums", "SC >>> Refresh Front Panel", "CURSOR >>> Default", "FP >>> Set User Level", "FP >>> Open"] ("State Queue OUT") w453 string[] ["CTRL >>> Signal Selector", "FP >>> Plot Active Curves", "FP >>> Plot Attributes", "FP >>> Window Title", "FP >>> Resize Panel", "CURSOR >>> Init Frequency Band"] ("State Queue OUT")] -> w445
          tunnel: [enum16{"Replace", "Append", "Prepend"}."Prepend" ("State Queue Options") enum16{"Replace", "Append", "Prepend"}."Prepend" ("State Queue Options") enum16{"Replace", "Append", "Prepend"}."Prepend" ("State Queue Options")] -> w444
          frame "Initialize", Default {
          }
          frame "Compute" {
            n210 = disable-structure shown="Disabled" {
              disable-tunnel: [w457 T10."Enabled" ("Disabled")] -> w452
              disable-tunnel: [w455 w463] -> w453
              frame Disabled {
                n211 = local read "Spectral Function Type"() -> (w456:T5)
                n212 = case shown="\"Auto Spectrum - (EU RMS)\", Default" w456 {
                  tunnel: [T10."Enabled" ("Disabled") T10."Disabled and Grayed Out" ("Disabled")] -> w457
                  tunnel: [w458 string[] ["SEND MSG >>> Computing Octave ...", "DP: Octave Band", "CLOSE MSG"]] -> w455
                  frame "Auto Spectrum - (EU RMS)", Default {
                    n213 = Build Array("DP: Process Spectrums" ("String")) -> (w458:string[])
                  }
                  frame "Auto Spectrum - (EU RMS)", "Auto Spectrum - (EU Peak)" {
                  }
                }
              }
              frame Enabled {
                n214 = Build Array("DP: Process Spectrums" ("String")) -> (w463:string[])
              }
            }
            n215 = property on="Spectral Function Parameters - User" class="Clust (strict)"("DisabledEnum"=w452) -> ()  [unwired: 2 in, 2 out]
          }
          frame "Refresh Front Panel" {
          }
        }
        n216 = call "Set State Queue.vi"("reference in"=w447, "error in (no error)"=w448, "State Queue Options"=w444, "State Queue"=w445) -> ("error out"=w446:errorcluster)  [unwired: 14 in, 1 out]
      }
      frame "---- Front Panel Mgmt ----" {
      }
      frame "FP" {
        n217 = case shown="\"Set User Level\"" w474 {
          selector: w474 -> [w477 _ _ _ _ _ _ _]
          tunnel: [w476 w480 w496 w529 w570 w595 w601 w638] -> w473
          tunnel: w472 -> [w476 w482 w494 w530 w571 w596 _ w638]
          tunnel: w471 -> [_ w481 w495 w531 w572 _ w602 _]
          tunnel: w470 -> [_ _ _ _ _ _ _ _]
          frame "False", Default {
            n218 = Concatenate Strings("The following FP command is unrecognized:\n" ("source"), w477) -> (w478:string)
            n219 = One Button Dialog(message=w478) -> ()  [unwired: 1 in, 1 out]
          }
          frame "Open" {
            n220 = call-dynamic "Get VI Ref.vi"("reference in"=w481, "error in (no error)"=w482) -> ("GUI VI Ref"=w487:refnum<vi>, "error out"=w486:errorcluster)  [unwired: 14 in, 2 out]
            n221 = property class="VI"(reference=w487, error in=w486) -> (reference out=w484:refnum<vi>, error out=w483:errorcluster, "Front Panel.Open"=w485:bool)
            n222 = case shown="False" w485 {
              tunnel: [w490 w493] -> w480
              tunnel: w483 -> [w489 w493]
              tunnel: w484 -> [w488 _]
              frame False {
                n223 = invoke class="VI" method="FP.Open"(reference=w488, error in=w489, "Activate"=TRUE, "State"=T11."Standard") -> (error out=w490:errorcluster)  [unwired: 1 in, 4 out]
              }
              frame True {
              }
            }
          }
          frame "Default Panel Position and Size" {
            (unwired) i16 5  # window border width
            (unwired) i16 31  # vertical Space from the top of the screen
            w516 = i16 0  # vertical Space from the top of the screen
            w513 = i16 28  # horizontal Space
            w511 = i16 625  # Default window width
            w510 = i16 660  # Default window height
            w509 = i16 31  # Space for the title bar and menu between each window
            w508 = i16 0  # window border width
            # "NOTE: This is the DEFAULT location AND size of the Panel"
            n224 = call "GetClass - Window Info.vi"("error in (no error)"=w494) -> ("Window Info"=w526:T17, "error out"=w527:errorcluster)  [unwired: 17 in]
            n225 = Open Application Reference(8:w527) -> (0:w504:errorcluster, 3:w506:refnum<vi>)  [unwired: 3 out]
            n226 = property class="App"(reference=w506, error in=w504) -> (reference out=w505:refnum<vi>, error out=w503:errorcluster, "Display:Primary Workspace"=w502:T19)
            n227 = Array Size(array=w526) -> (size(s)=w507:i32)
            n228 = Decrement(x=w507) -> (x-1=w517:i32)
            n229 = To Word Integer(number=w517) -> (16bit integer=w514:i16)
            n230 = Unbundle By Name(w502) -> ("Right"=w520:i16, "Left"=w521:i16)
            n231 = Close Reference(reference=w505, error in (no error)=w503) -> (error out=w523:errorcluster)
            n232 = Multiply(x=w514, y=w509) -> (x*y=w515:i16)
            n233 = Subtract(x=w520, y=w521) -> (x-y=w522:i16)
            n234 = To Word Integer(number=w522) -> (16bit integer=w519:i16)
            n235 = Subtract(x=w519, y=w508) -> (x-y=w518:i16)
            n236 = call-dynamic "Get VI Ref.vi"("reference in"=w495, "error in (no error)"=w523) -> ("GUI VI Ref"=w525:refnum<vi>, "error out"=w524:errorcluster)  [unwired: 14 in, 2 out]
            n237 = Multiply(x=w513, y=w514) -> (x*y=w512:i16)
            n238 = Subtract(x=w518, y=w512) -> (x-y=w500:i16)
            n239 = Subtract(x=w500, y=w511) -> (x-y=w498:i16)
            n240 = Add(x=w515, y=w516) -> (x+y=w499:i16)
            n241 = Add(x=w499, y=w510) -> (x+y=w501:i16)
            n242 = Bundle By Name(cluster=w502, "Left"=w498, "Top"=w499, "Right"=w500, "Bottom"=w501) -> (w497:T19)
            n243 = property class="VI"(reference=w525, error in=w524, "Front Panel.WinBounds"=w497) -> (error out=w496:errorcluster)  [unwired: 1 out]
          }
          frame "Resize Panel" {
            w546 = i16 660  # Default Height
            # "Bug in LabView that generates an error on the FP.Winbounds if the scroll bar is ALWAYS ON??"
            # "The Panel is resize base on the number of channels"
            n244 = call "Get - Data Obj.vi"("reference in"=w531, "error in (no error)"=w530) -> ("reference out"=w561:refnum<class "gSPWB.lvclass">, "Data"=w562:refnum<class "GSwFormDSP.lvclass">, "error out"=w563:errorcluster)  [unwired: 15 in]
            n245 = call-dynamic "Get - Nb wForms.vi"("reference in"=w562, "error in (no error)"=w563) -> ("Nb Wave Forms"=w558:i32, "error out"=w559:errorcluster)  [unwired: 15 in, 1 out]
            n246 = Less?(x=w558, y=17 ("x")) -> (x < y?=w538:bool)
            n247 = case shown="False" w538 {
              tunnel: [16 w569] -> w548
              tunnel: w558 -> [_ w569]
              tunnel: [w564 T12."Off While Running" ("Vertical Scrollbar Visibility")] -> w536
              frame False {
                n248 = disable-structure shown="Disabled" {
                  disable-tunnel: [T12."Always On" ("Vertical Scrollbar Visibility") T12."Off While Running" ("Vertical Scrollbar Visibility")] -> w564
                  frame Disabled {
                  }
                  frame Enabled {
                  }
                }
              }
              frame True {
              }
            }
            n249 = call-dynamic "Get VI Ref.vi"("reference in"=w561, "error in (no error)"=w559) -> ("GUI VI Ref"=w557:refnum<vi>, "error out"=w556:errorcluster)  [unwired: 14 in, 2 out]
            n250 = property class="VI"(reference=w557, error in=w556) -> (reference out=w560:refnum<vi>, error out=w554:errorcluster, "Panel"=w553:refnum<vi>, "Front Panel.WinBounds"=w532:T19)
            n251 = property class="Pnl"(reference=w553, error in=w554) -> (error out=w555:errorcluster, "Panes[]"=w551:refnum<vi>[])  [unwired: 1 out]
            n252 = Subtract(x=w548, y=6) -> (x-y=w540:i32)
            n253 = Multiply(x=w540, y=24) -> (x*y=w542:i32)
            n254 = To Word Integer(number=w542) -> (16bit integer=w544:i16)
            n255 = Index Array(array=w551, index=0) -> (element=w550:refnum<vi>)
            n256 = Unbundle By Name(w532) -> ("Top"=w547:i16)
            n257 = Greater Than 0?(x=w544) -> (x > 0?=w543:bool)
            n258 = property class="Pane"(reference=w550, error in=w555, "VertScrollbarVisibility"=w536) -> (error out=w528:errorcluster)  [unwired: 1 out]
            n259 = Add(x=w547, y=w546) -> (x+y=w535:i16)
            n260 = Select(t=w544, s=w543, f=i16 0) -> (s? t:f=w534:i16)
            n261 = Add(x=w535, y=w534) -> (x+y=w549:i16)
            n262 = Bundle By Name(cluster=w532, "Bottom"=w549) -> (w533:T19)
            n263 = property class="VI"(reference=w560, error in=w528, "Front Panel.WinBounds"=w533) -> (error out=w529:errorcluster)  [unwired: 1 out]
          }
          frame "Window Title" {
            n264 = call "Get - Data Obj.vi"("reference in"=w572, "error in (no error)"=w571) -> ("reference out"=w577:refnum<class "gSPWB.lvclass">, "Data"=w582:refnum<class "GSwFormDSP.lvclass">, "error out"=w583:errorcluster)  [unwired: 15 in]
            n265 = call-dynamic "Get - Paths.vi"("reference in"=w582, "error in (no error)"=w583) -> ("Nb Different Paths"=w585:i32, "Path Names"=w584:string[], "error out"=w586:errorcluster)  [unwired: 14 in, 1 out]
            n266 = case shown="0, 1" w585 {
              tunnel: w584 -> [_ w593]
              tunnel: ["Multiple data source" ("Output String") w589] -> w574
              frame 2, Default {
              }
              frame 0, 1 {
                # "Assumes they all have the same filenames"
                n267 = Index Array(array=w593) -> (element=w591:string)  [unwired: 1 in]
                n268 = String To Path(string=w591) -> (path=w592:path)
                n269 = call "Truncate full path to a given string length.vi"("Max. Number of allowable characters"=55, "Truncation Option"=T13."Keep the full path - Force file name display", "Full Path"=w592) -> ("Output String"=w589:string)  [unwired: 8 in]
              }
            }
            n270 = call "Get - Window Name Index.vi"("reference in"=w577, "error in (no error)"=w586) -> ("Window Name Index"=w579:string, "reference out"=w578:refnum<class "gSPWB.lvclass">, "error out"=w581:errorcluster)  [unwired: 15 in]
            n271 = call-dynamic "Get VI Ref.vi"("reference in"=w578, "error in (no error)"=w581) -> ("GUI VI Ref"=w576:refnum<vi>, "error out"=w575:errorcluster)  [unwired: 14 in, 2 out]
            n272 = Concatenate Strings(w579, ": " ("string"), w574) -> (w580:string)
            n273 = property class="VI"(reference=w576, error in=w575, "Front Panel.Title"=w580) -> (error out=w570:errorcluster)  [unwired: 1 out]
          }
          frame "Plot Active Curves" {
            n274 = for {
              shift-right: [w598] -> w595
              shift-left: w596 -> [w600]
              tunnel: "Signals selector" -> [w597] mode=indexing
              i -> [w599]
              n275 = property on="Graph" class="WFGraph (strict)"(error in=w600, "Active Plot"=w599, "Plot.Visible?"=w597) -> (error out=w598:errorcluster)  [unwired: 1 in, 1 out]
            }
          }
          frame "Plot Attributes" {
            n276 = property on="Graph" class="WFGraph (strict)"() -> (error out=w605:errorcluster, "Label.Text"=w604:string)  [unwired: 2 in, 1 out]
            n277 = local read "Signals selector"() -> (w606:bool[])
            n278 = Array Size(array=w606) -> (size(s)=w603:i32)
            n279 = for {
              N: w603 -> [_]
              shift-right: [w616] -> w601
              shift-left: w605 -> [w611]
              tunnel: w604 -> [w610]
              tunnel: w602 -> [w612]
              i -> [w613]
              n280 = Number To Decimal String(number=w613) -> (decimal integer string=w614:string)  [unwired: 1 in]
              n281 = Concatenate Strings("Plot " ("string"), w614) -> (w609:string)
              n282 = call-dynamic "Read Default Values from Disk.vi"("reference in"=w612, "error in (no error)"=w611, "Control Label"=w610, "Caption"=w609) -> ("Value (XML String)"=w607:string, "error out"=w608:errorcluster)  [unwired: 13 in, 1 out]
              n283 = case shown="\"ALL\", Default" w607 {
                selector: w607 -> [w634 _]
                tunnel: [w636 w637] -> w616
                tunnel: w608 -> [w635 w637]
                tunnel: w613 -> [w632 _]
                frame "ALL", Default {
                  n284 = Unflatten From XML(xml string=w634, type=T14 {"Color"=0, "PointStyle"=0, "LineStyle"=0, "Interp"=0, "LineWidth"=0, "BarPlotStyle"=0, "FillTo"=0, "XScaleIdx"=0, "YScaleIdx"=0, "Anti-Aliased"=FALSE, "LabelFormat"=0, "TransitionType"=0, "TransitionLocation"=0, "DigitalLineStyle"=0} ("Template Att."), error in (no error)=w635) -> (value=w620:T14, error out=w633:errorcluster)
                  n285 = Unbundle By Name(w620) -> ("Color"=w631:u32, "PointStyle"=w630:u8, "LineStyle"=w629:u8, "Interp"=w628:u8, "LineWidth"=w627:u8, "BarPlotStyle"=w626:u8, "FillTo"=w625:i16, "XScaleIdx"=w624:u32, "YScaleIdx"=w623:u32, "LabelFormat"=w622:u8, "TransitionType"=w621:u8, "TransitionLocation"=w619:u8, "DigitalLineStyle"=w618:u8)  [unwired: 1 out]
                  n286 = property on="Graph" class="WFGraph (strict)"(error in=w633, "Active Plot"=w632, "Plot.Plot Color"=w631, "Plot.Point Style"=w630, "Plot.Line Style"=w629, "Plot.Plot Interpolation"=w628, "Plot.Line Width"=w627, "Plot.Bar Plot Style"=w626, "Plot.Fill To"=w625, "Plot.XScaleIdx"=w624, "Plot.YScaleIdx"=w623, "Plot.Label Style"=w622, "Plot.Transition Type"=w621, "Plot.TransitionLocation"=w619, "Plot.DigitalLineStyle"=w618) -> (error out=w636:errorcluster)  [unwired: 1 in, 1 out]
                }
                frame "" {
                }
              }
            }
          }
          frame "Set User Level" {
          }
        }
      }
      frame "CTRL" {
        n287 = case shown="\"Version Number\"" w641 {
          selector: w641 -> [w647 _ _ _ _ _ _ _]
          tunnel: [w645 w651 w675 w691 w702 w705 w746 w796] -> w643
          tunnel: w642 -> [w645 w656 w677 w693 w703 w706 w745 w798]
          tunnel: w640 -> [_ w661 w673 w689 _ w707 w744 w799]
          tunnel: w639 -> [_ _ _ _ _ _ w747 _]
          frame "unknown", Default {
            n288 = Concatenate Strings("The Following Control identifier is unrecognized:\n" ("source"), w647) -> (w646:string)
            n289 = One Button Dialog(message=w646) -> ()  [unwired: 1 in, 1 out]
          }
          frame "Spectral Function Parameters" {
            n290 = property on="Spectral Function Parameters - User" class="Clust (strict)"(error in=w656) -> (error out=w655:errorcluster, "Label.Text"=w654:string, "Value"=w653:T7)  [unwired: 1 in, 1 out]
            n291 = call-dynamic "Read Default Values from Disk.vi"("reference in"=w661, "error in (no error)"=w655, "Control Label"=w654) -> ("Value (XML String)"=w649:string, "reference out"=w657:refnum<class "SPWB.lvclass">, "error out"=w658:errorcluster)  [unwired: 14 in]
            n292 = Empty String/Path?(string/path=w649) -> (empty?=w662:bool)
            n293 = case shown="False" w662 {
              tunnel: [w665 w668] -> w650
              tunnel: w649 -> [w664 _]
              tunnel: w653 -> [w663 w668]
              frame False {
                n294 = Unflatten From XML(xml string=w664, type=w663) -> (value=w666:T7, error out=w667:errorcluster)  [unwired: 1 in]
                n295 = Select(t=w663, s=w667, f=w666) -> (s? t:f=w665:T7)
              }
              frame True {
              }
            }
            n296 = call "Get - Data Obj.vi"("reference in"=w657, "error in (no error)"=w658) -> ("Data"=w660:refnum<class "GSwFormDSP.lvclass">, "error out"=w659:errorcluster)  [unwired: 15 in, 1 out]
            n297 = call "Set FFT - Spectral Parameters.vi"("reference in"=w660, "error in (no error)"=w659, "Spectral Function Parameters - User"=w650) -> ("error out"=w652:errorcluster)  [unwired: 15 in, 1 out]
            n298 = property on="Spectral Function Parameters - User" class="Clust (strict)"(error in=w652, "Value"=w650) -> (error out=w651:errorcluster)  [unwired: 1 in, 1 out]
          }
          frame "Spectral Function Type" {
            n299 = property on="Spectral Function Type" class="Enum (strict)"(error in=w677) -> (error out=w672:errorcluster, "Label.Text"=w671:string, "Value"=w676:T5)  [unwired: 1 in, 1 out]
            n300 = call-dynamic "Read Default Values from Disk.vi"("reference in"=w673, "error in (no error)"=w672, "Control Label"=w671) -> ("Value (XML String)"=w669:string, "error out"=w670:errorcluster)  [unwired: 14 in, 1 out]
            n301 = Empty String/Path?(string/path=w669) -> (empty?=w678:bool)
            n302 = case shown="False" w678 {
              tunnel: [w681 w684] -> w674
              tunnel: w669 -> [w680 _]
              tunnel: w676 -> [w679 w684]
              frame False {
                n303 = Unflatten From XML(xml string=w680, type=w679) -> (value=w682:T5, error out=w683:errorcluster)  [unwired: 1 in]
                n304 = Select(t=w679, s=w683, f=w682) -> (s? t:f=w681:T5)
              }
              frame True {
              }
            }
            n305 = property on="Spectral Function Type" class="Enum (strict)"(error in=w670, "Value"=w674) -> (error out=w675:errorcluster)  [unwired: 1 in, 1 out]
          }
          frame "Spectrum Display Options" {
            n306 = property on="Spectrum Display Options" class="Enum (strict)"(error in=w693) -> (error out=w688:errorcluster, "Label.Text"=w687:string, "Value"=w692:T4)  [unwired: 1 in, 1 out]
            n307 = call-dynamic "Read Default Values from Disk.vi"("reference in"=w689, "error in (no error)"=w688, "Control Label"=w687) -> ("Value (XML String)"=w685:string, "error out"=w686:errorcluster)  [unwired: 14 in, 1 out]
            n308 = Empty String/Path?(string/path=w685) -> (empty?=w694:bool)
            n309 = case shown="False" w694 {
              tunnel: [w697 w700] -> w690
              tunnel: w685 -> [w696 _]
              tunnel: w692 -> [w695 w700]
              frame False {
                n310 = Unflatten From XML(xml string=w696, type=w695) -> (value=w698:T4, error out=w699:errorcluster)  [unwired: 1 in]
                n311 = Select(t=w695, s=w699, f=w698) -> (s? t:f=w697:T4)
              }
              frame True {
              }
            }
            n312 = property on="Spectrum Display Options" class="Enum (strict)"(error in=w686, "Value"=w690) -> (error out=w691:errorcluster)  [unwired: 1 in, 1 out]
          }
          frame "DSP Function" {
            n313 = property on="DSP Functions" class="TabCtl (strict)"(error in=w703, "Value"=T1."Spectral Analysis" ("DSP Functions")) -> (error out=w702:errorcluster)  [unwired: 1 in, 1 out]
          }
          frame "Signal Selector" {
            n314 = call "Get - Data Obj.vi"("reference in"=w707, "error in (no error)"=w706) -> ("Data"=w709:refnum<class "GSwFormDSP.lvclass">, "error out"=w710:errorcluster)  [unwired: 15 in, 1 out]
            n315 = call-dynamic "Get - Nb wForms.vi"("reference in"=w709, "error in (no error)"=w710) -> ("Nb Wave Forms"=w704:i32, "error out"=w708:errorcluster)  [unwired: 15 in, 1 out]
            n316 = Equal To 0?(x=w704) -> (x = 0?=w741:bool)
            n317 = Select(t=1, s=w741, f=w704) -> (s? t:f=w730:i32)
            n318 = To Double Precision Float(number=w730) -> (double precision float=w735:dbl)
            n319 = property on="Graph" class="WFGraph (strict)"(error in=w708) -> (error out=w732:errorcluster, "LegTop"=w726:i32, "LegLeft"=w724:i32, "LegWidth"=w723:u32, "LegHt"=w733:u32)  [unwired: 1 in, 1 out]
            n320 = To Double Precision Float(number=w733) -> (double precision float=w734:dbl)
            n321 = Divide(x=w734, y=w735) -> (x/y=w740:dbl)
            n322 = Initialize Array(TRUE, w730) -> (w731:bool[])
            n323 = Multiply(x=w740, y=1.0) -> (x*y=w739:dbl)
            n324 = To Long Integer(number=w723) -> (32bit integer=w722:i32)
            n325 = Multiply(x=w740, y=0.675) -> (x*y=w737:dbl)
            n326 = To Unsigned Long Integer(number=w739) -> (unsigned 32bit integer=w715:u32)
            n327 = Add(x=w724, y=w722) -> (x+y=w729:i32)
            n328 = To Unsigned Long Integer(number=w737) -> (unsigned 32bit integer=w717:u32)
            n329 = To Unsigned Long Integer(number=w730) -> (unsigned 32bit integer=w720:u32)
            n330 = Subtract(x=w726, y=3) -> (x-y=w725:i32)
            n331 = Subtract(x=w729, y=30) -> (x-y=w721:i32)
            n332 = control-ref of="String"() -> (w714:refnum<vi>)
            n333 = property on="Signals selector" class="Arr (strict)"(error in=w732, "Value"=w731, "Number of Rows"=w720, "Top"=w725, "Left"=w721) -> (error out=w713:errorcluster, "Array Element"=w716:refnum<vi>)  [unwired: 1 in, 1 out]
            n334 = To More Specific Class(target class=refnum<vi> refnum ("Boolean 2"), reference=w716, error in=w713) -> (specific class reference=w719:refnum<vi>, error out=w712:errorcluster)
            n335 = property class="Bool (strict)"(reference=w719, error in=w712, "Height"=w717) -> (error out=w711:errorcluster)  [unwired: 1 out]
            n336 = property class="Str"(reference=w714, error in=w711, "Height"=w715) -> (error out=w705:errorcluster)  [unwired: 1 out]
          }
          frame "Start - End Freq Band" {
            n337 = case shown="\"Read\"" w747 {
              selector: w747 -> [w749 _ _]
              tunnel: [w748 w754 w783] -> w746
              tunnel: w745 -> [w748 w764 w792]
              tunnel: w744 -> [_ w763 w790]
              frame "", Default {
                n338 = Concatenate Strings("The Following \"CTRL >>> Start-End Freq Band >>\" identifier is unrecognized:\n" ("source"), w749) -> (w750:string)
                n339 = One Button Dialog(message=w750) -> ()  [unwired: 1 in, 1 out]
              }
              frame "Read" {
                n340 = property on="Start Frequency (Hz)" class="DigNum (strict)"(error in=w764) -> (error out=w767:errorcluster, "Label.Text"=w766:string, "Value"=w769:dbl)  [unwired: 1 in, 1 out]
                n341 = call-dynamic "Read Default Values from Disk.vi"("reference in"=w763, "error in (no error)"=w767, "Control Label"=w766) -> ("Value (XML String)"=w753:string, "reference out"=w756:refnum<class "SPWB.lvclass">, "error out"=w765:errorcluster)  [unwired: 14 in]
                n342 = Empty String/Path?(string/path=w753) -> (empty?=w770:bool)
                n343 = case shown="False" w770 {
                  tunnel: [w779 w782] -> w768
                  tunnel: w753 -> [w778 _]
                  tunnel: w769 -> [w777 w782]
                  frame False {
                    n344 = Unflatten From XML(xml string=w778, type=w777) -> (value=w780:dbl, error out=w781:errorcluster)  [unwired: 1 in]
                    n345 = Select(t=w777, s=w781, f=w780) -> (s? t:f=w779:dbl)
                  }
                  frame True {
                  }
                }
                n346 = property on="Start Frequency (Hz)" class="DigNum (strict)"(error in=w765, "Value"=w768) -> (error out=w755:errorcluster)  [unwired: 1 in, 1 out]
                n347 = property on="End Frequency (Hz)" class="DigNum (strict)"(error in=w755) -> (error out=w760:errorcluster, "Label.Text"=w761:string, "Value"=w758:dbl)  [unwired: 1 in, 1 out]
                n348 = call-dynamic "Read Default Values from Disk.vi"("reference in"=w756, "error in (no error)"=w760, "Control Label"=w761) -> ("Value (XML String)"=w752:string, "error out"=w762:errorcluster)  [unwired: 14 in, 1 out]
                n349 = Empty String/Path?(string/path=w752) -> (empty?=w757:bool)
                n350 = case shown="False" w757 {
                  tunnel: [w773 w776] -> w759
                  tunnel: w752 -> [w772 _]
                  tunnel: w758 -> [w771 w776]
                  frame False {
                    n351 = Unflatten From XML(xml string=w772, type=w771) -> (value=w774:dbl, error out=w775:errorcluster)  [unwired: 1 in]
                    n352 = Select(t=w771, s=w775, f=w774) -> (s? t:f=w773:dbl)
                  }
                  frame True {
                  }
                }
                n353 = property on="End Frequency (Hz)" class="DigNum (strict)"(error in=w762, "Value"=w759) -> (error out=w754:errorcluster)  [unwired: 1 in, 1 out]
              }
              frame "Write" {
                n354 = property on="Start Frequency (Hz)" class="DigNum (strict)"(error in=w792) -> (error out=w795:errorcluster, "Label.Text"=w794:string, "Value"=w791:dbl)  [unwired: 1 in, 1 out]
                n355 = Flatten To XML(6:w791) -> (2:w793:string)
                n356 = call-dynamic "Write Default Values to disk.vi"("reference in"=w790, "error in (no error)"=w795, "Control Label"=w794, "Value (XML String)"=w793) -> ("reference out"=w784:refnum<class "SPWB.lvclass">, "error out"=w785:errorcluster)  [unwired: 14 in]
                n357 = property on="End Frequency (Hz)" class="DigNum (strict)"(error in=w785) -> (error out=w786:errorcluster, "Label.Text"=w787:string, "Value"=w789:dbl)  [unwired: 1 in, 1 out]
                n358 = Flatten To XML(6:w789) -> (2:w788:string)
                n359 = call-dynamic "Write Default Values to disk.vi"("reference in"=w784, "error in (no error)"=w786, "Control Label"=w787, "Value (XML String)"=w788) -> ("error out"=w783:errorcluster)  [unwired: 14 in, 1 out]
              }
            }
          }
          frame "Version Number" {
            n360 = call "Get Version Number.vi"("reference in"=w799, "error in (no error)"=w798) -> ("Version #"=→"Version":string, "error out"=w796:errorcluster)  [unwired: 15 in, 1 out]
          }
        }
      }
      frame "CURSOR" {
        n361 = case shown="\"Frequency Band\"" w800 {
          selector: w800 -> [w805 _ _ _]
          tunnel: [w804 w818 w820 w833] -> w802
          tunnel: w801 -> [w804 w813 w821 w834]
          frame "False", Default {
            n362 = Concatenate Strings("The following CURSOR state is unrecognized:\n" ("source"), w805) -> (w806:string)
            n363 = One Button Dialog(message=w806) -> ()  [unwired: 1 in, 1 out]
          }
          frame "Default" {
            # "Only keep the first cursor"
            n364 = property on="Graph" class="WFGraph (strict)"(error in=w813) -> (error out=w814:errorcluster, "CrsrList"=w812:T15)  [unwired: 1 in, 1 out]
            n365 = Index Array(array=w812) -> (element=w811:T16)  [unwired: 1 in]
            n366 = Bundle By Name(cluster=w811, "Name"="Cursor", "Plot"=0, "Cursor Mode"=u32 1, "Watch All Plots"=TRUE) -> (w816:T16)
            n367 = Build Array(w816) -> (w815:T20)
            n368 = property on="Graph" class="WFGraph (strict)"(error in=w814, "CrsrList"=w815) -> (error out=w818:errorcluster)  [unwired: 1 in, 1 out]
          }
          frame "Frequency Band" {
            n369 = local read "Start Frequency (Hz)"() -> (w819:dbl)
            n370 = local read "End Frequency (Hz)"() -> (w832:dbl)
            n371 = property on="Graph" class="WFGraph (strict)"(error in=w821) -> (error out=w829:errorcluster, "CrsrList"=w828:T15)  [unwired: 1 in, 1 out]
            n372 = Index Array(array=w828) -> (element=w827:T16)  [unwired: 1 in]
            n373 = Bundle By Name(cluster=w827, "Name"="Start", "Plot"=-1, "Cursor Mode"=u32 1, "Position.X"=w819) -> (w826:T16)
            n374 = Bundle By Name(cluster=w826, "Name"="End", "Position.X"=w832) -> (w824:T16)
            n375 = Build Array(w826, w824) -> (w830:T20)
            n376 = property on="Graph" class="WFGraph (strict)"(error in=w829, "CrsrList"=w830) -> (error out=w820:errorcluster)  [unwired: 1 in, 1 out]
          }
          frame "Init Frequency Band" {
            # "This sets up the controls for the energy band computation."
            n377 = local read "PSD"() -> (w836:waveform(dbl)[])
            n378 = for {
              tunnel: w836 -> [w862] mode=indexing
              tunnel: [w858] -> w839 mode=indexing
              tunnel: [w856] -> w838 mode=indexing
              n379 = Unbundle By Name(w862) -> ("Y"=w861:dbl[], "dt"=w856:dbl)
              n380 = Array Size(array=w861) -> (size(s)=w860:i32)
              n381 = Decrement(x=w860) -> (x-1=w857:i32)
              n382 = To Double Precision Float(number=w857) -> (double precision float=w859:dbl)
              n383 = Multiply(x=w859, y=w856) -> (x*y=w858:dbl)
            }
            n384 = Array Max & Min(array=w839) -> (max value=w835:dbl)  [unwired: 3 out]
            n385 = Array Max & Min(array=w838) -> (min value=w837:dbl)  [unwired: 3 out]
            n386 = disable-structure shown="Enabled" {
              disable-tunnel: w837 -> [w846 w854]
              disable-tunnel: w835 -> [w844 w852]
              disable-tunnel: w834 -> [w841 w849]
              disable-tunnel: [w840 w848] -> w833
              frame Disabled {
                w847 = 0.0 ("Start Frequency (Hz)")
                n387 = Round Toward -Infinity(1:w844) -> (0:w842:dbl)
                n388 = property on="Start Frequency (Hz)" class="DigNum (strict)"(error in=w841, "Maximum"=w842, "Increment"=w846, "Minimum"=w847, "Value"=w847) -> (error out=w843:errorcluster)  [unwired: 1 in, 1 out]
                n389 = local write "End Frequency (Hz)"(w842) -> ()
                n390 = property on="End Frequency (Hz)" class="DigNum (strict)"(error in=w843, "Maximum"=w842, "Increment"=w846, "Minimum"=0.0 ("Start Frequency (Hz)"), "Value"=w842) -> (error out=w840:errorcluster)  [unwired: 1 in, 1 out]
              }
              frame Enabled {
                n391 = Round Toward -Infinity(1:w852) -> (0:w850:dbl)
                n392 = property on="Start Frequency (Hz)" class="DigNum (strict)"(error in=w849, "Maximum"=w850, "Increment"=w854, "Minimum"=0.0 ("Start Frequency (Hz)")) -> (error out=w851:errorcluster)  [unwired: 1 in, 1 out]
                n393 = property on="End Frequency (Hz)" class="DigNum (strict)"(error in=w851, "Maximum"=w850, "Increment"=w854, "Minimum"=0.0 ("Start Frequency (Hz)")) -> (error out=w848:errorcluster)  [unwired: 1 in, 1 out]
              }
            }
          }
        }
      }
      frame "---- GUI Functions ----" {
      }
      frame "GUI: Initialize Ref" {
        # "Must WRITE Back the Object so the new reference is saved!"
        n394 = control-ref of="GUI Reference"() -> (w881:refnum<vi>)
        n395 = call "Set VI Ref.vi"("reference in"=w879, "error in (no error)"=w880, "ReInit All to Default?"=FALSE, "GUI VI Ref"=w881, "Initialize FP Control Refs"=TRUE) -> ("reference out"=w882:refnum<class "SPWB.lvclass">, "error out"=w884:errorcluster)  [unwired: 13 in]
        n396 = call "Set Close Panel (Yes or No).vi"("reference in"=w882, "error in (no error)"=w884) -> ("reference out"=w883:refnum<class "SPWB.lvclass">, "error out"=w885:errorcluster)  [unwired: 16 in]
        n397 = call "Set Message Window Ref.vi"("reference in"=w883, "error in (no error)"=w885) -> ("reference out"=w888:refnum<class "SPWB.lvclass">, "error out"=w889:errorcluster)  [unwired: 16 in]
        n398 = call "Get - Data Obj.vi"("reference in"=w888, "error in (no error)"=w889) -> ("reference out"=w874:refnum<class "gSPWB.lvclass">, "Data"=w873:refnum<class "GSwFormDSP.lvclass">, "error out"=w872:errorcluster)  [unwired: 15 in]
        n399 = call "Set - wForms.vi"("reference in"=w873, "error in (no error)"=w872, "Init wForms"=TRUE, "wForms"="wForms") -> ("reference out"=w868:refnum<class "GSwFormDSP.lvclass">, "error out"=w875:errorcluster)  [unwired: 14 in]
        n400 = call "Set - Data Obj.vi"("reference in"=w874, "Data"=w868, "error in (no error)"=w875) -> ("reference out"=w869:refnum<class "gSPWB.lvclass">, "error out"=w870:errorcluster)  [unwired: 15 in]
        n401 = call "Get - Window Name Index.vi"("reference in"=w869, "error in (no error)"=w870) -> ("Window Name Index"=w890:string, "error out"=w886:errorcluster)  [unwired: 15 in, 1 out]
        n402 = call "GetClass - Window Info.vi"("error in (no error)"=w886) -> ("Window Info"=w878:T17, "error out"=w887:errorcluster)  [unwired: 17 in]
        n403 = Bundle("Window Name Index"=w890, "reference out"=w868) -> (w891:T21)  [unwired: 1 in]
        n404 = Build Array (concatenate)(w878, w891) -> (w877:T22)
        n405 = call "SetClass - Window Info.vi"("error in (no error)"=w887, "Window Info"=w877) -> ("error out"=w876:errorcluster)  [unwired: 17 in]
      }
      frame "GUI: Exit" {
        # "If it is the last window, NEED to run the garbage collector"
        n406 = call "Get - Window Name Index.vi"("reference in"=w895, "error in (no error)"=w894) -> ("Window Name Index"=w912:string, "reference out"=w909:refnum<class "gSPWB.lvclass">, "error out"=w910:errorcluster)  [unwired: 15 in]
        n407 = call-dynamic "Get Message Window Ref.vi"("reference in"=w909, "error in (no error)"=w910) -> ("reference out"=w906:refnum<class "gSPWB.lvclass">, "Msg Win Ref"=w908:refnum<vi>, "error out"=w907:errorcluster)  [unwired: 15 in]
        n408 = call-dynamic "Get VI Ref.vi"("reference in"=w906, "error in (no error)"=w907) -> ("reference out"=w902:refnum<class "gSPWB.lvclass">, "GUI VI Ref"=w904:refnum<vi>, "error out"=w903:errorcluster)  [unwired: 14 in, 1 out]
        n409 = call-dynamic "Get Close Panel (Yes or No).vi"("reference in"=w902, "error in (no error)"=w903) -> ("Close Panel?"=w901:bool, "reference out"=w899:refnum<class "gSPWB.lvclass">, "error out"=w900:errorcluster)  [unwired: 15 in]
        n410 = call-dynamic "Destroy.vi"("reference in"=w899, "error in (no error)"=w900) -> ("error out"=w911:errorcluster)  [unwired: 16 in, 1 out]
        n411 = call "GetClass - Window Info.vi"("error in (no error)"=w911) -> ("Window Info"=w919:T17, "error out"=w914:errorcluster)  [unwired: 17 in]
        n412 = for {
          tunnel: w919 -> [w923] mode=indexing
          tunnel: [w922] -> w920 mode=indexing
          n413 = Unbundle By Name(w923) -> ("Window Name Index"=w922:string)
        }
        n414 = Search 1D Array(1D array=w920, element=w912) -> (index of element=w918:i32)  [unwired: 1 in]
        n415 = Delete From Array(array=w919, length=1, index=w918) -> (array with subset deleted=w915)  [unwired: 1 out]
        n416 = call "SetClass - Window Info.vi"("error in (no error)"=w914, "Window Info"=w915) -> ("error out"=w917:errorcluster)  [unwired: 17 in]
        n417 = Empty Array?(array=w915) -> (empty?=w916:bool)
        n418 = case shown="True" w916 {
          tunnel: [w924 w926] -> w905
          tunnel: w917 -> [w924 w925]
          frame False {
          }
          frame True {
            n419 = call <vilib>:"GarbageCollector.vi"("error in (no error)"=w925) -> ("error out"=w926:errorcluster)  [unwired: 16 in, 2 out]
          }
        }
        n420 = Close Reference(reference=w908, error in (no error)=w905) -> (error out=w896:errorcluster)
        n421 = case shown="True" w901 {
          tunnel: w896 -> [w928 w932]
          tunnel: [w928 w931] -> w898
          tunnel: [w927 w930] -> w897
          tunnel: w904 -> [w927 w929]
          frame False {
          }
          frame True {
            n422 = property class="VI"(reference=w929, error in=w932) -> (reference out=w934:refnum<vi>, error out=w933:errorcluster, "Front Panel.Open"=w935:bool)
            n423 = case shown="True" w935 {
              tunnel: [w937 w941] -> w931
              tunnel: w933 -> [w937 w940]
              tunnel: w934 -> [w936 w939]
              tunnel: [w936 w938] -> w930
              frame False {
              }
              frame True {
                n424 = invoke class="VI" method="FP.Close"(reference=w939, error in=w940) -> (reference out=w938:refnum<vi>, error out=w941:errorcluster)  [unwired: 1 in, 1 out]
              }
            }
          }
        }
        n425 = Close Reference(reference=w897, error in (no error)=w898) -> (error out=w893:errorcluster)
      }
      frame "SEND MSG" {
        n426 = call-dynamic "Get Message Window Ref.vi"("reference in"=w944, "error in (no error)"=w943) -> ("Msg Win Ref"=w955:refnum<vi>, "error out"=w954:errorcluster)  [unwired: 15 in, 1 out]
        n427 = property class="VI"(reference=w955, error in=w954) -> (reference out=w952:refnum<vi>, error out=w953:errorcluster, "Front Panel.Open"=w951:bool)
        n428 = case shown="False" w951 {
          tunnel: [w963 w967] -> w949
          tunnel: w953 -> [w958 w967]
          tunnel: w952 -> [w960 w966]
          tunnel: [w962 w966] -> w950
          frame False {
            w961 = FALSE ("Wait Until Done")
            n429 = invoke class="VI" method="Run VI"(reference=w960, error in=w958, "Wait until done"=w961, "Auto Dispose Ref"=w961) -> (reference out=w959:refnum<vi>, error out=w957:errorcluster)  [unwired: 1 in, 3 out]
            n430 = invoke class="VI" method="FP.Open"(reference=w959, error in=w957, "Activate"=TRUE, "State"=T11."Standard") -> (reference out=w962:refnum<vi>, error out=w963:errorcluster)  [unwired: 1 in, 3 out]
          }
          frame True {
          }
        }
        n431 = Concatenate Strings("\r\n", w945) -> (w946:string)
        n432 = invoke class="VI" method="Ctrl Val.Set"(reference=w950, error in=w949, "Control Name"="Message", "Value"=w946) -> (error out=w942:errorcluster)  [unwired: 1 in, 4 out]
      }
      frame "CLOSE MSG" {
        n433 = call-dynamic "Get Message Window Ref.vi"("reference in"=w969, "error in (no error)"=w970) -> ("Msg Win Ref"=w977:refnum<vi>, "error out"=w976:errorcluster)  [unwired: 15 in, 1 out]
        n434 = property class="VI"(reference=w977, error in=w976) -> (reference out=w972:refnum<vi>, error out=w971:errorcluster, "Front Panel.Open"=w973:bool)
        n435 = case shown="True" w973 {
          tunnel: [w980 w984] -> w974
          tunnel: w971 -> [w980 w983]
          tunnel: w972 -> [w979 w982]
          tunnel: [w979 w981] -> w975
          frame False {
          }
          frame True {
            n436 = invoke class="VI" method="FP.Close"(reference=w982, error in=w983) -> (reference out=w981:refnum<vi>, error out=w984:errorcluster)  [unwired: 1 in, 1 out]
          }
        }
        n437 = invoke class="VI" method="Abort VI"(reference=w975, error in=w974) -> (error out=w968:errorcluster)  [unwired: 1 in, 2 out]
      }
      frame "---- Miscelleneous ----" {
      }
      frame "unknown", Default {
        n438 = Concatenate Strings("The following state is unrecognized?\n", w989) -> (w987:string)
        n439 = One Button Dialog(message=w987) -> ()  [unwired: 1 in, 1 out]
      }
      frame "Error" {
        w994 = "\r"
        # "Clears the error"
        n440 = Array Size(array=w1000) -> (size(s)=w1003:i32)
        n441 = Decrement(x=w1003) -> (x-1=w1002:i32)
        n442 = Unbundle By Name(w997) -> ("source"=w1004:string)
        n443 = Decrement(x=w1002) -> (x-1=w1001:i32)
        n444 = Index Array(array=w1000, index #1=w1001) -> (element #1=w999:string, element #2=w992:string)  [unwired: 1 in]
        n445 = Concatenate Strings(w1004, w994, "Before last State: " ("string"), w999, w994, "Last State: " ("string"), w992) -> (w996:string)
        n446 = Bundle By Name(cluster=w997, "source"=w996) -> (w995:errorcluster)
        n447 = call <vilib>:"General Error Handler.vi"("error in (no error)"=w995) -> ()  [unwired: 10 in, 5 out]
      }
      frame "Next" {
        # "This is an empty case used so the queue does NOT stop if there is an empty string between two valid states!"
      }
      frame "Quit" {
        n448 = flat-sequence {
          frame #0 {
            n449 = One Button Dialog(message="The state machine has crashed!  The software will now close!") -> ()  [unwired: 1 in, 1 out]
          }
          frame #1 {
            n450 = control-ref of="This VI"() -> (w1014:refnum<vi>)
            n451 = invoke class="VI" method="FP.Close"(reference=w1014) -> (reference out=w1012:refnum<vi>, error out=w1013:errorcluster)  [unwired: 2 in, 1 out]
            n452 = Close Reference(reference=w1012, error in (no error)=w1013) -> ()  [unwired: 1 out]
          }
        }
      }
    }
  }
